vi "NernstIV.vi"() -> ()   [LabVIEW 2020]
uses:
  <userlib>/LevyLab/LV-Data/LV-Data/Typedefs/Dictionary--cluster.ctl
  <userlib>/LevyLab/LV-Data/LV-Data/Typedefs/File Type--enum.ctl
  <userlib>/LevyLab/XY Utilities/subVIs/Subtract XY (single).vi
  <userlib>/LevyLab/XY Utilities/subVIs/Moving Average (single).vi
  <userlib>/LevyLab/XY Utilities/subVIs/Get X and Y (single).vi
  <userlib>/LevyLab/XY Utilities/Private/X Units.vi
  <userlib>/LevyLab/XY Utilities/Private/X Array Range to Index.vi
  <userlib>/_OpenG.lib/array/array.llb/Sort Array__ogtk.vi
  <userlib>/_OpenG.lib/array/array.llb/Sort 1D Array (DBL)__ogtk.vi
  <userlib>/_OpenG.lib/array/array.llb/Reorder Array2__ogtk.vi
  <userlib>/_OpenG.lib/array/array.llb/Reorder 1D Array2 (DBL)__ogtk.vi
  <vilib>/ptbypt/Probability & Statistics.llb/Mean PtByPt.vi
  <vilib>/Utility/error.llb/Error Cluster From Error Code.vi
  <userlib>/LevyLab/LV-Data/LV-Data/LV-Data.lvclass
  <userlib>/LevyLab/XY Utilities/xy_utilities.lvlib
panel:
  in  "Avg Window":dbl
  out "Error vs Temp 2T":cluster{dbl[], dbl[]}[](graph)=[{[0.099648], [2.4953013324737623e-06]}]
  in  "Antisym?":bool
  in  "length per file":i32=196
  in  "index":i32=99
  out "Error vs Temp":cluster{dbl[], dbl[]}[](graph)=[{[0.099648], [0.0]}]
  in  "File Type":T1=enum."TDMS"
  out "counter":i32
  out "Path":path=path "G:/.shortcut-targets-by-id/0B8-gGFa6hkR4XzJJMDlqZXVKRk0/ansom/Data/PPMS 3/SA40511C.20250205/08-IVWire1nd2_heating/SA40511C.20250205.000008.tdms"
  out "Comments":string="Device: \r  Device Name: SA40511C.20250205\r  Computer: PPMS3DAQ\r  User: Ranjani\r  Instrument: PPMS 3\r  Description: |\r    LAO/KTO 3wire Nernst\r\rExperiment: \r  Time: 2025-02-08T20:02:05\r  Description: |\r    T =100mK\r    B= 1T\r    \r    I1 and 2+= 0 to -50m to 50m to 0V, 30s\r    wait, 2s\r    I+/- = 2/5\r    V+/- = 1/26\r    I2+/- = 3/4\r    Wire 3\r    I3+/- =100 mV @13Hz (346nA)\r\rSweep: \r- Loop1: [OFF, 0.000000]\r- Loop2: [OFF, 0.000000]\r- Loop3: [OFF, 0.000000]\r- Loop4: [OFF, 0.000000]\r\rWiring: \r- Electrode 1: Lockin 1, V1+\r- Electrode 2: Lockin 2, I+\r- Electrode 3: Lockin 3, I2+\r- Electrode 4: Lockin 4, I2-\r- Electrode 5: Lockin 5, I-\r- Electrode 26: Lockin 6, V1-\r- Electrode 27: Lockin 7, I3+\r- Electrode 28: Lockin 8, I3+\r\rLockin: \r  AO: \r  - AO 1: amp = 0.000 mV, DC = 0.000 mV, f = 13.00 Hz, phi = 0.00°, Sine\r  - AO 2: amp = 0.000 mV, DC = 0.001 mV, f = 13.00 Hz, phi = 0.00°, Sine\r  - AO 3: amp = 0.000 mV, DC = 0.001 mV, f = 13.00 Hz, phi = 0.00°, Sine\r  - AO 4: amp = 0.000 mV, DC = 0.000 mV, f = 13.00 Hz, phi = 0.00°, Sine\r  - AO 5: amp = 0.000 mV, DC = 0.000 mV, f = 13.00 Hz, phi = 0.00°, Sine\r  - AO 6: amp = 0.000 mV, DC = 0.000 mV, f = 13.00 Hz, phi = 0.00°, Sine\r  - AO 7: amp = 0.000 mV, DC = 0.000 mV, f = 13.00 Hz, phi = 0.00°, Sine\r  - AO 8: amp = 100.000 mV, DC = 0.000 mV, f = 13.00 Hz, phi = 0.00°, Sine\r  REF: \r  - Lockin 1: f = 13.00 Hz, phi = 0.00°, TC = 0.10 s, order = 2 \r  - Lockin 2: f = 26.00 Hz, phi = 0.00°, TC = 0.10 s, order = 2 \r  Sampling: \r  - Fs: 13000.000000\r  - N: 1000\r"
  in  "index":T2={"I+(A)"="AO2", "I-(A)"="AI5", "V4T+"="AI1", "V4T-"="AI6", "UG"="AO3", "DG"="AO4", "LG"="AO8", "B"="Magnet", "Temperature"="Temperature", "Vfast"="Temperature", "Vslow"="Magnet"}
  in  "SE?":bool=TRUE
  out "Data (Dictionary)":T3[](array[typedef])=[{"key"="Time", "value"=variant(dbl[] [3821910664.275333])}, {"key"="Temperature", "value"=variant(dbl[] [0.099648])}, {"key"="Magnet", "value"=variant(dbl[] [0.99993349609375])}, {"key"="AO1", "value"=variant(dbl[] [0.0, 0.0, 0.0, 0.0, 0.0, 0.0, 0.0, 0.0, 0.0, 0.0, 0.0, 0.0, 0.0, 0.0, 0.0, 0.0, 0.0, 0.0, 0.0, 0.0, 0.0, 0.0, 0.0, 0.0, 0.0, 0.0, 0.0, 0.0, 0.0, 0.0, 0.0, 0.0, 0.0, 0.0, 0.0, 0.0, 0.0, 0.0, 0.0, 0.0, 0.0, 0.0, 0.0, 0.0, 0.0, 0.0, 0.0, 0.0, 0.0, 0.0, 0.0, 0.0, 0.0, 0.0, 0.0, 0.0, 0.0, 0.0, 0.0, 0.0, 0.0, 0.0, 0.0, 0.0, 0.0, 0.0, 0.0, 0.0, 0.0, 0.0, 0.0, 0.0, 0.0, 0.0, 0.0, 0.0, 0.0, 0.0, 0.0, 0.0, 0.0, 0.0, 0.0, 0.0, 0.0, 0.0, 0.0, 0.0, 0.0, 0.0, 0.0, 0.0, 0.0, 0.0, 0.0, 0.0, 0.0, 0.0, 0.0, 0.0, 0.0, 0.0, 0.0, 0.0, 0.0, 0.0, 0.0, 0.0, 0.0, 0.0, 0.0, 0.0, 0.0, 0.0, 0.0, 0.0, 0.0, 0.0, 0.0, 0.0, 0.0, 0.0, 0.0, 0.0, 0.0, 0.0, 0.0, 0.0, 0.0, 0.0, 0.0, 0.0, 0.0, 0.0, 0.0, 0.0, 0.0, 0.0, 0.0, 0.0, 0.0, 0.0, 0.0, 0.0, 0.0, 0.0, 0.0, 0.0, 0.0, 0.0, 0.0, 0.0, 0.0, 0.0, 0.0, 0.0, 0.0, 0.0, 0.0, 0.0, 0.0, 0.0, 0.0, 0.0, 0.0, 0.0, 0.0, 0.0, 0.0, 0.0, 0.0, 0.0, 0.0, 0.0, 0.0, 0.0, 0.0, 0.0, 0.0, 0.0, 0.0, 0.0, 0.0, 0.0, 0.0, 0.0, 0.0, 0.0, 0.0, 0.0, 0.0, 0.0, 0.0, 0.0, 0.0, 0.0, 0.0, 0.0, 0.0, 0.0, 0.0, 0.0, 0.0, 0.0, 0.0, 0.0, 0.0, 0.0, 0.0, 0.0, 0.0, 0.0, 0.0, 0.0, 0.0, 0.0, 0.0, 0.0, 0.0, 0.0, 0.0, 0.0, 0.0, 0.0, 0.0, 0.0, 0.0, 0.0, 0.0, 0.0, 0.0, 0.0, 0.0, 0.0, 0.0, 0.0, 0.0, 0.0, 0.0, 0.0, 0.0, 0.0, 0.0, 0.0, 0.0, 0.0, 0.0, 0.0, 0.0, 0.0, 0.0, 0.0, 0.0, 0.0, 0.0, 0.0, 0.0, 0.0, 0.0, 0.0, 0.0, 0.0, 0.0, 0.0, 0.0, 0.0, 0.0, 0.0, 0.0, 0.0, 0.0, 0.0, 0.0, 0.0, 0.0, 0.0, 0.0, 0.0, 0.0, 0.0, 0.0, 0.0, 0.0, 0.0, 0.0, 0.0, 0.0, 0.0, 0.0, 0.0, 0.0, 0.0, 0.0, 0.0, 0.0, 0.0, 0.0, 0.0, 0.0, 0.0, 0.0, 0.0, 0.0, 0.0, 0.0, 0.0, 0.0, 0.0, 0.0, 0.0, 0.0, 0.0, 0.0, 0.0, 0.0, 0.0, 0.0, 0.0, 0.0, 0.0, 0.0, 0.0, 0.0, 0.0, 0.0, 0.0, 0.0, 0.0, 0.0, 0.0, 0.0, 0.0, 0.0, 0.0, 0.0, 0.0, 0.0, 0.0, 0.0, 0.0, 0.0, 0.0, 0.0, 0.0, 0.0, 0.0, 0.0, 0.0, 0.0, 0.0, 0.0, 0.0, 0.0, 0.0, 0.0, 0.0, 0.0, 0.0, 0.0, 0.0, 0.0, 0.0, 0.0, 0.0, 0.0, 0.0, 0.0, 0.0, 0.0, 0.0, 0.0, 0.0, 0.0, 0.0, 0.0, 0.0, 0.0, 0.0, 0.0, 0.0, 0.0, 0.0, 0.0, 0.0, 0.0, 0.0, 0.0, 0.0, 0.0, 0.0])}, {"key"="AO2", "value"=variant(dbl[] array[390 elements])}, {"key"="AO3", "value"=variant(dbl[] array[390 elements])}, {"key"="AO4", "value"=variant(dbl[] [0.0, 0.0, 0.0, 0.0, 0.0, 0.0, 0.0, 0.0, 0.0, 0.0, 0.0, 0.0, 0.0, 0.0, 0.0, 0.0, 0.0, 0.0, 0.0, 0.0, 0.0, 0.0, 0.0, 0.0, 0.0, 0.0, 0.0, 0.0, 0.0, 0.0, 0.0, 0.0, 0.0, 0.0, 0.0, 0.0, 0.0, 0.0, 0.0, 0.0, 0.0, 0.0, 0.0, 0.0, 0.0, 0.0, 0.0, 0.0, 0.0, 0.0, 0.0, 0.0, 0.0, 0.0, 0.0, 0.0, 0.0, 0.0, 0.0, 0.0, 0.0, 0.0, 0.0, 0.0, 0.0, 0.0, 0.0, 0.0, 0.0, 0.0, 0.0, 0.0, 0.0, 0.0, 0.0, 0.0, 0.0, 0.0, 0.0, 0.0, 0.0, 0.0, 0.0, 0.0, 0.0, 0.0, 0.0, 0.0, 0.0, 0.0, 0.0, 0.0, 0.0, 0.0, 0.0, 0.0, 0.0, 0.0, 0.0, 0.0, 0.0, 0.0, 0.0, 0.0, 0.0, 0.0, 0.0, 0.0, 0.0, 0.0, 0.0, 0.0, 0.0, 0.0, 0.0, 0.0, 0.0, 0.0, 0.0, 0.0, 0.0, 0.0, 0.0, 0.0, 0.0, 0.0, 0.0, 0.0, 0.0, 0.0, 0.0, 0.0, 0.0, 0.0, 0.0, 0.0, 0.0, 0.0, 0.0, 0.0, 0.0, 0.0, 0.0, 0.0, 0.0, 0.0, 0.0, 0.0, 0.0, 0.0, 0.0, 0.0, 0.0, 0.0, 0.0, 0.0, 0.0, 0.0, 0.0, 0.0, 0.0, 0.0, 0.0, 0.0, 0.0, 0.0, 0.0, 0.0, 0.0, 0.0, 0.0, 0.0, 0.0, 0.0, 0.0, 0.0, 0.0, 0.0, 0.0, 0.0, 0.0, 0.0, 0.0, 0.0, 0.0, 0.0, 0.0, 0.0, 0.0, 0.0, 0.0, 0.0, 0.0, 0.0, 0.0, 0.0, 0.0, 0.0, 0.0, 0.0, 0.0, 0.0, 0.0, 0.0, 0.0, 0.0, 0.0, 0.0, 0.0, 0.0, 0.0, 0.0, 0.0, 0.0, 0.0, 0.0, 0.0, 0.0, 0.0, 0.0, 0.0, 0.0, 0.0, 0.0, 0.0, 0.0, 0.0, 0.0, 0.0, 0.0, 0.0, 0.0, 0.0, 0.0, 0.0, 0.0, 0.0, 0.0, 0.0, 0.0, 0.0, 0.0, 0.0, 0.0, 0.0, 0.0, 0.0, 0.0, 0.0, 0.0, 0.0, 0.0, 0.0, 0.0, 0.0, 0.0, 0.0, 0.0, 0.0, 0.0, 0.0, 0.0, 0.0, 0.0, 0.0, 0.0, 0.0, 0.0, 0.0, 0.0, 0.0, 0.0, 0.0, 0.0, 0.0, 0.0, 0.0, 0.0, 0.0, 0.0, 0.0, 0.0, 0.0, 0.0, 0.0, 0.0, 0.0, 0.0, 0.0, 0.0, 0.0, 0.0, 0.0, 0.0, 0.0, 0.0, 0.0, 0.0, 0.0, 0.0, 0.0, 0.0, 0.0, 0.0, 0.0, 0.0, 0.0, 0.0, 0.0, 0.0, 0.0, 0.0, 0.0, 0.0, 0.0, 0.0, 0.0, 0.0, 0.0, 0.0, 0.0, 0.0, 0.0, 0.0, 0.0, 0.0, 0.0, 0.0, 0.0, 0.0, 0.0, 0.0, 0.0, 0.0, 0.0, 0.0, 0.0, 0.0, 0.0, 0.0, 0.0, 0.0, 0.0, 0.0, 0.0, 0.0, 0.0, 0.0, 0.0, 0.0, 0.0, 0.0, 0.0, 0.0, 0.0, 0.0, 0.0, 0.0, 0.0, 0.0, 0.0, 0.0, 0.0, 0.0, 0.0, 0.0, 0.0, 0.0, 0.0, 0.0, 0.0, 0.0, 0.0, 0.0, 0.0, 0.0, 0.0, 0.0, 0.0, 0.0, 0.0, 0.0, 0.0, 0.0, 0.0, 0.0, 0.0, 0.0, 0.0, 0.0])}, {"key"="AO5", "value"=variant(dbl[] [0.0, 0.0, 0.0, 0.0, 0.0, 0.0, 0.0, 0.0, 0.0, 0.0, 0.0, 0.0, 0.0, 0.0, 0.0, 0.0, 0.0, 0.0, 0.0, 0.0, 0.0, 0.0, 0.0, 0.0, 0.0, 0.0, 0.0, 0.0, 0.0, 0.0, 0.0, 0.0, 0.0, 0.0, 0.0, 0.0, 0.0, 0.0, 0.0, 0.0, 0.0, 0.0, 0.0, 0.0, 0.0, 0.0, 0.0, 0.0, 0.0, 0.0, 0.0, 0.0, 0.0, 0.0, 0.0, 0.0, 0.0, 0.0, 0.0, 0.0, 0.0, 0.0, 0.0, 0.0, 0.0, 0.0, 0.0, 0.0, 0.0, 0.0, 0.0, 0.0, 0.0, 0.0, 0.0, 0.0, 0.0, 0.0, 0.0, 0.0, 0.0, 0.0, 0.0, 0.0, 0.0, 0.0, 0.0, 0.0, 0.0, 0.0, 0.0, 0.0, 0.0, 0.0, 0.0, 0.0, 0.0, 0.0, 0.0, 0.0, 0.0, 0.0, 0.0, 0.0, 0.0, 0.0, 0.0, 0.0, 0.0, 0.0, 0.0, 0.0, 0.0, 0.0, 0.0, 0.0, 0.0, 0.0, 0.0, 0.0, 0.0, 0.0, 0.0, 0.0, 0.0, 0.0, 0.0, 0.0, 0.0, 0.0, 0.0, 0.0, 0.0, 0.0, 0.0, 0.0, 0.0, 0.0, 0.0, 0.0, 0.0, 0.0, 0.0, 0.0, 0.0, 0.0, 0.0, 0.0, 0.0, 0.0, 0.0, 0.0, 0.0, 0.0, 0.0, 0.0, 0.0, 0.0, 0.0, 0.0, 0.0, 0.0, 0.0, 0.0, 0.0, 0.0, 0.0, 0.0, 0.0, 0.0, 0.0, 0.0, 0.0, 0.0, 0.0, 0.0, 0.0, 0.0, 0.0, 0.0, 0.0, 0.0, 0.0, 0.0, 0.0, 0.0, 0.0, 0.0, 0.0, 0.0, 0.0, 0.0, 0.0, 0.0, 0.0, 0.0, 0.0, 0.0, 0.0, 0.0, 0.0, 0.0, 0.0, 0.0, 0.0, 0.0, 0.0, 0.0, 0.0, 0.0, 0.0, 0.0, 0.0, 0.0, 0.0, 0.0, 0.0, 0.0, 0.0, 0.0, 0.0, 0.0, 0.0, 0.0, 0.0, 0.0, 0.0, 0.0, 0.0, 0.0, 0.0, 0.0, 0.0, 0.0, 0.0, 0.0, 0.0, 0.0, 0.0, 0.0, 0.0, 0.0, 0.0, 0.0, 0.0, 0.0, 0.0, 0.0, 0.0, 0.0, 0.0, 0.0, 0.0, 0.0, 0.0, 0.0, 0.0, 0.0, 0.0, 0.0, 0.0, 0.0, 0.0, 0.0, 0.0, 0.0, 0.0, 0.0, 0.0, 0.0, 0.0, 0.0, 0.0, 0.0, 0.0, 0.0, 0.0, 0.0, 0.0, 0.0, 0.0, 0.0, 0.0, 0.0, 0.0, 0.0, 0.0, 0.0, 0.0, 0.0, 0.0, 0.0, 0.0, 0.0, 0.0, 0.0, 0.0, 0.0, 0.0, 0.0, 0.0, 0.0, 0.0, 0.0, 0.0, 0.0, 0.0, 0.0, 0.0, 0.0, 0.0, 0.0, 0.0, 0.0, 0.0, 0.0, 0.0, 0.0, 0.0, 0.0, 0.0, 0.0, 0.0, 0.0, 0.0, 0.0, 0.0, 0.0, 0.0, 0.0, 0.0, 0.0, 0.0, 0.0, 0.0, 0.0, 0.0, 0.0, 0.0, 0.0, 0.0, 0.0, 0.0, 0.0, 0.0, 0.0, 0.0, 0.0, 0.0, 0.0, 0.0, 0.0, 0.0, 0.0, 0.0, 0.0, 0.0, 0.0, 0.0, 0.0, 0.0, 0.0, 0.0, 0.0, 0.0, 0.0, 0.0, 0.0, 0.0, 0.0, 0.0, 0.0, 0.0, 0.0, 0.0, 0.0, 0.0, 0.0, 0.0, 0.0, 0.0, 0.0, 0.0, 0.0, 0.0, 0.0, 0.0, 0.0, 0.0, 0.0])}, {"key"="AO6", "value"=variant(dbl[] [0.0, 0.0, 0.0, 0.0, 0.0, 0.0, 0.0, 0.0, 0.0, 0.0, 0.0, 0.0, 0.0, 0.0, 0.0, 0.0, 0.0, 0.0, 0.0, 0.0, 0.0, 0.0, 0.0, 0.0, 0.0, 0.0, 0.0, 0.0, 0.0, 0.0, 0.0, 0.0, 0.0, 0.0, 0.0, 0.0, 0.0, 0.0, 0.0, 0.0, 0.0, 0.0, 0.0, 0.0, 0.0, 0.0, 0.0, 0.0, 0.0, 0.0, 0.0, 0.0, 0.0, 0.0, 0.0, 0.0, 0.0, 0.0, 0.0, 0.0, 0.0, 0.0, 0.0, 0.0, 0.0, 0.0, 0.0, 0.0, 0.0, 0.0, 0.0, 0.0, 0.0, 0.0, 0.0, 0.0, 0.0, 0.0, 0.0, 0.0, 0.0, 0.0, 0.0, 0.0, 0.0, 0.0, 0.0, 0.0, 0.0, 0.0, 0.0, 0.0, 0.0, 0.0, 0.0, 0.0, 0.0, 0.0, 0.0, 0.0, 0.0, 0.0, 0.0, 0.0, 0.0, 0.0, 0.0, 0.0, 0.0, 0.0, 0.0, 0.0, 0.0, 0.0, 0.0, 0.0, 0.0, 0.0, 0.0, 0.0, 0.0, 0.0, 0.0, 0.0, 0.0, 0.0, 0.0, 0.0, 0.0, 0.0, 0.0, 0.0, 0.0, 0.0, 0.0, 0.0, 0.0, 0.0, 0.0, 0.0, 0.0, 0.0, 0.0, 0.0, 0.0, 0.0, 0.0, 0.0, 0.0, 0.0, 0.0, 0.0, 0.0, 0.0, 0.0, 0.0, 0.0, 0.0, 0.0, 0.0, 0.0, 0.0, 0.0, 0.0, 0.0, 0.0, 0.0, 0.0, 0.0, 0.0, 0.0, 0.0, 0.0, 0.0, 0.0, 0.0, 0.0, 0.0, 0.0, 0.0, 0.0, 0.0, 0.0, 0.0, 0.0, 0.0, 0.0, 0.0, 0.0, 0.0, 0.0, 0.0, 0.0, 0.0, 0.0, 0.0, 0.0, 0.0, 0.0, 0.0, 0.0, 0.0, 0.0, 0.0, 0.0, 0.0, 0.0, 0.0, 0.0, 0.0, 0.0, 0.0, 0.0, 0.0, 0.0, 0.0, 0.0, 0.0, 0.0, 0.0, 0.0, 0.0, 0.0, 0.0, 0.0, 0.0, 0.0, 0.0, 0.0, 0.0, 0.0, 0.0, 0.0, 0.0, 0.0, 0.0, 0.0, 0.0, 0.0, 0.0, 0.0, 0.0, 0.0, 0.0, 0.0, 0.0, 0.0, 0.0, 0.0, 0.0, 0.0, 0.0, 0.0, 0.0, 0.0, 0.0, 0.0, 0.0, 0.0, 0.0, 0.0, 0.0, 0.0, 0.0, 0.0, 0.0, 0.0, 0.0, 0.0, 0.0, 0.0, 0.0, 0.0, 0.0, 0.0, 0.0, 0.0, 0.0, 0.0, 0.0, 0.0, 0.0, 0.0, 0.0, 0.0, 0.0, 0.0, 0.0, 0.0, 0.0, 0.0, 0.0, 0.0, 0.0, 0.0, 0.0, 0.0, 0.0, 0.0, 0.0, 0.0, 0.0, 0.0, 0.0, 0.0, 0.0, 0.0, 0.0, 0.0, 0.0, 0.0, 0.0, 0.0, 0.0, 0.0, 0.0, 0.0, 0.0, 0.0, 0.0, 0.0, 0.0, 0.0, 0.0, 0.0, 0.0, 0.0, 0.0, 0.0, 0.0, 0.0, 0.0, 0.0, 0.0, 0.0, 0.0, 0.0, 0.0, 0.0, 0.0, 0.0, 0.0, 0.0, 0.0, 0.0, 0.0, 0.0, 0.0, 0.0, 0.0, 0.0, 0.0, 0.0, 0.0, 0.0, 0.0, 0.0, 0.0, 0.0, 0.0, 0.0, 0.0, 0.0, 0.0, 0.0, 0.0, 0.0, 0.0, 0.0, 0.0, 0.0, 0.0, 0.0, 0.0, 0.0, 0.0, 0.0, 0.0, 0.0, 0.0, 0.0, 0.0, 0.0, 0.0, 0.0, 0.0, 0.0, 0.0, 0.0, 0.0])}, {"key"="AO7", "value"=variant(dbl[] [0.0, 0.0, 0.0, 0.0, 0.0, 0.0, 0.0, 0.0, 0.0, 0.0, 0.0, 0.0, 0.0, 0.0, 0.0, 0.0, 0.0, 0.0, 0.0, 0.0, 0.0, 0.0, 0.0, 0.0, 0.0, 0.0, 0.0, 0.0, 0.0, 0.0, 0.0, 0.0, 0.0, 0.0, 0.0, 0.0, 0.0, 0.0, 0.0, 0.0, 0.0, 0.0, 0.0, 0.0, 0.0, 0.0, 0.0, 0.0, 0.0, 0.0, 0.0, 0.0, 0.0, 0.0, 0.0, 0.0, 0.0, 0.0, 0.0, 0.0, 0.0, 0.0, 0.0, 0.0, 0.0, 0.0, 0.0, 0.0, 0.0, 0.0, 0.0, 0.0, 0.0, 0.0, 0.0, 0.0, 0.0, 0.0, 0.0, 0.0, 0.0, 0.0, 0.0, 0.0, 0.0, 0.0, 0.0, 0.0, 0.0, 0.0, 0.0, 0.0, 0.0, 0.0, 0.0, 0.0, 0.0, 0.0, 0.0, 0.0, 0.0, 0.0, 0.0, 0.0, 0.0, 0.0, 0.0, 0.0, 0.0, 0.0, 0.0, 0.0, 0.0, 0.0, 0.0, 0.0, 0.0, 0.0, 0.0, 0.0, 0.0, 0.0, 0.0, 0.0, 0.0, 0.0, 0.0, 0.0, 0.0, 0.0, 0.0, 0.0, 0.0, 0.0, 0.0, 0.0, 0.0, 0.0, 0.0, 0.0, 0.0, 0.0, 0.0, 0.0, 0.0, 0.0, 0.0, 0.0, 0.0, 0.0, 0.0, 0.0, 0.0, 0.0, 0.0, 0.0, 0.0, 0.0, 0.0, 0.0, 0.0, 0.0, 0.0, 0.0, 0.0, 0.0, 0.0, 0.0, 0.0, 0.0, 0.0, 0.0, 0.0, 0.0, 0.0, 0.0, 0.0, 0.0, 0.0, 0.0, 0.0, 0.0, 0.0, 0.0, 0.0, 0.0, 0.0, 0.0, 0.0, 0.0, 0.0, 0.0, 0.0, 0.0, 0.0, 0.0, 0.0, 0.0, 0.0, 0.0, 0.0, 0.0, 0.0, 0.0, 0.0, 0.0, 0.0, 0.0, 0.0, 0.0, 0.0, 0.0, 0.0, 0.0, 0.0, 0.0, 0.0, 0.0, 0.0, 0.0, 0.0, 0.0, 0.0, 0.0, 0.0, 0.0, 0.0, 0.0, 0.0, 0.0, 0.0, 0.0, 0.0, 0.0, 0.0, 0.0, 0.0, 0.0, 0.0, 0.0, 0.0, 0.0, 0.0, 0.0, 0.0, 0.0, 0.0, 0.0, 0.0, 0.0, 0.0, 0.0, 0.0, 0.0, 0.0, 0.0, 0.0, 0.0, 0.0, 0.0, 0.0, 0.0, 0.0, 0.0, 0.0, 0.0, 0.0, 0.0, 0.0, 0.0, 0.0, 0.0, 0.0, 0.0, 0.0, 0.0, 0.0, 0.0, 0.0, 0.0, 0.0, 0.0, 0.0, 0.0, 0.0, 0.0, 0.0, 0.0, 0.0, 0.0, 0.0, 0.0, 0.0, 0.0, 0.0, 0.0, 0.0, 0.0, 0.0, 0.0, 0.0, 0.0, 0.0, 0.0, 0.0, 0.0, 0.0, 0.0, 0.0, 0.0, 0.0, 0.0, 0.0, 0.0, 0.0, 0.0, 0.0, 0.0, 0.0, 0.0, 0.0, 0.0, 0.0, 0.0, 0.0, 0.0, 0.0, 0.0, 0.0, 0.0, 0.0, 0.0, 0.0, 0.0, 0.0, 0.0, 0.0, 0.0, 0.0, 0.0, 0.0, 0.0, 0.0, 0.0, 0.0, 0.0, 0.0, 0.0, 0.0, 0.0, 0.0, 0.0, 0.0, 0.0, 0.0, 0.0, 0.0, 0.0, 0.0, 0.0, 0.0, 0.0, 0.0, 0.0, 0.0, 0.0, 0.0, 0.0, 0.0, 0.0, 0.0, 0.0, 0.0, 0.0, 0.0, 0.0, 0.0, 0.0, 0.0, 0.0, 0.0, 0.0, 0.0, 0.0, 0.0, 0.0, 0.0, 0.0, 0.0, 0.0])}, {"key"="AO8", "value"=variant(dbl[] array[390 elements])}, {"key"="AI1", "value"=variant(dbl[] array[390 elements])}, {"key"="AI2", "value"=variant(dbl[] array[390 elements])}, {"key"="AI3", "value"=variant(dbl[] array[390 elements])}, {"key"="AI4", "value"=variant(dbl[] array[390 elements])}, {"key"="AI5", "value"=variant(dbl[] array[390 elements])}, {"key"="AI6", "value"=variant(dbl[] array[390 elements])}, {"key"="AI7", "value"=variant(dbl[] array[390 elements])}, {"key"="AI8", "value"=variant(dbl[] array[390 elements])}, {"key"="X1", "value"=variant(dbl[] array[390 elements])}, {"key"="X2", "value"=variant(dbl[] array[390 elements])}, {"key"="X3", "value"=variant(dbl[] array[390 elements])}, {"key"="X4", "value"=variant(dbl[] array[390 elements])}, {"key"="X5", "value"=variant(dbl[] array[390 elements])}, {"key"="X6", "value"=variant(dbl[] array[390 elements])}, {"key"="X7", "value"=variant(dbl[] array[390 elements])}, {"key"="X8", "value"=variant(dbl[] array[390 elements])}, {"key"="Y1", "value"=variant(dbl[] array[390 elements])}, {"key"="Y2", "value"=variant(dbl[] array[390 elements])}, {"key"="Y3", "value"=variant(dbl[] array[390 elements])}, {"key"="Y4", "value"=variant(dbl[] array[390 elements])}, {"key"="Y5", "value"=variant(dbl[] array[390 elements])}, {"key"="Y6", "value"=variant(dbl[] array[390 elements])}, {"key"="Y7", "value"=variant(dbl[] array[390 elements])}, {"key"="Y8", "value"=variant(dbl[] array[390 elements])}]
  out "Gates, B and T":T4={"UG"=-0.000255897435897436, "DG"=0.0, "LG"=7.77808822991638e-13, "B"=0.99993349609375, "Temperature"=0.099648}
  in  "Subtract from 4T":cluster{dbl[], dbl[]}[](graph)=[{[-0.020298805594444295, -0.020143332123756498, -0.019935172677040203, -0.019711892008781505, -0.019499069094658004, -0.019296326518058897, -0.0190861269235612, -0.018870721936226, -0.0186526147127153, -0.0184441012144091, -0.018240182995796404, -0.018026167988777403, -0.017805154204368796, -0.0175968400239946, -0.017388032078743197, -0.017181379437446798, -0.016960291981697302, -0.016742527604103302, -0.0165384343862536, -0.0163279012441638, -0.0161165035963061, -0.0158924008607867, -0.0156821869611742, -0.015477146983146901, -0.015263935208320902, -0.0150432082414629, -0.014828914046287701, -0.0146212004423143, -0.0144141832590105, -0.0141964107751848, -0.0139734686613085, -0.013768090128898802, -0.0135563558340074, -0.013346166729927202, -0.013120899081230299, -0.0129057987928392, -0.012701104283332999, -0.012487238287925912, -0.01226870453357717, -0.01204702484607715, -0.01183656013011947, -0.01162859666347524, -0.01141238462924974, -0.01118832433223746, -0.010975580811500699, -0.01076415216922773, -0.010553850293159662, -0.010330365061760138, -0.010109158396721092, -0.009902112841606301, -0.00968768084049235, -0.00947194325923932, -0.009244939923286621, -0.009032684683799868, -0.00882454001903547, -0.00860845100879677, -0.00838605582714088, -0.008168872952461409, -0.00795692384243022, -0.007747506260871981, -0.007525480151176509, -0.007301862120628491, -0.007093491911888181, -0.0068792678117752595, -0.0066681920289994095, -0.00644138252735143, -0.0062280436754227, -0.00602158486843118, -0.005808955550193789, -0.00559199845790865, -0.00537080562114718, -0.005163264632225051, -0.0049578579664230306, -0.00474451506137847, -0.004523096442222571, -0.004317351222038229, -0.0041118384599685195, -0.0039091233015059994, -0.00369388210773464, -0.0034842001199722, -0.0032883435487746897, -0.0030877457857131797, -0.0028865646123886, -0.0026763523817062403, -0.00248287928104402, -0.0022957037687301902, -0.0021012431383133304, -0.0018998574018478898, -0.00170761549472813, -0.0015246480703354297, -0.0013457845449447899, -0.0011569598913192998, -0.0009671784639358609, -0.000797939419746412, -0.0006248732805252139, -0.00045578753948211396, -0.00027331769466399497, -0.00010534942150116299, 4.9853920936584e-05, 0.00021248924732208502, 0.00038257944583893004, 0.000559727311134333, 0.000726794123649592, 0.000892312169075, 0.00107245266437529, 0.0012648783922195202, 0.00144211494922634, 0.00162198793888088, 0.0018035722970962, 0.00200244796276088, 0.0021988219022750504, 0.0023840004205703496, 0.00257733285427093, 0.0027730993032455404, 0.00298340857028962, 0.00318200647830965, 0.0033764384984970304, 0.00358172023296359, 0.0037975507974625003, 0.00400608170032506, 0.004211035609245349, 0.00441424405574801, 0.00463290369510651, 0.004853630900382989, 0.00505880463123321, 0.00527102982997892, 0.00548183524608609, 0.00570913612842555, 0.0059262028932570805, 0.0061337746381759, 0.006350606799125561, 0.00657308328151695, 0.006797502160072209, 0.00701170980930318, 0.007223751902580171, 0.007445839762687629, 0.0076745249032973495, 0.00788892495632163, 0.008105991482734609, 0.00832066643238058, 0.00854929745197286, 0.008773327469825608, 0.008985962748527383, 0.009204881548881421, 0.00942662870883931, 0.009656422495841838, 0.009873687624931172, 0.01008750140666952, 0.010308032870292512, 0.010535851359367219, 0.010755051493644521, 0.01097254836559275, 0.011186535954475272, 0.01141592419147475, 0.01164573872089373, 0.01185890591144548, 0.01207890450954417, 0.01229698598384842, 0.0125287271738051, 0.012748497128486448, 0.012961129307746701, 0.0131815141439436, 0.0134082280397413, 0.013634177565574501, 0.0138529192209242, 0.014067153573036, 0.014290386795997399, 0.0145212532281873, 0.0147375079393385, 0.014956275105476199, 0.015173210740089201, 0.0154038113355635, 0.0156266974210737, 0.0158396693468092, 0.016059869408607298, 0.0162831009626387, 0.0165129681825636, 0.0167303055524824, 0.016944220423698197, 0.0171680797338483, 0.0173991161584852, 0.017618041872978, 0.017834319472312697, 0.018048580527305402, 0.0182773231267927, 0.018506924033164802, 0.0187209612131117, 0.018940549969673003, 0.0191605340242385, 0.019393757939338598, 0.019613784909248304, 0.0198268069028853, 0.0200480521917343, 0.020275678992271395, 0.0205016232728957, 0.0206638196706772], [-1.88530516624451e-07, -1.87133288383484e-07, -1.85253167152405e-07, -1.83320441246033e-07, -1.81518726348877e-07, -1.79542255401611e-07, -1.77687950134277e-07, -1.75797801017761e-07, -1.73898572921753e-07, -1.71995229721069e-07, -1.70092630386353e-07, -1.68203616142273e-07, -1.6635901927948e-07, -1.64455137252808e-07, -1.62550988197327e-07, -1.60638189315796e-07, -1.58735628128052e-07, -1.56911063194275e-07, -1.54978852272034e-07, -1.53096804618836e-07, -1.51216950416565e-07, -1.49291834831238e-07, -1.47456007003784e-07, -1.45557689666748e-07, -1.4364326953888e-07, -1.41811571121216e-07, -1.3987343788147e-07, -1.38007555007935e-07, -1.36112055778503e-07, -1.34210629463196e-07, -1.3238597869873e-07, -1.30467686653137e-07, -1.28578906059265e-07, -1.26701898574829e-07, -1.24821209907532e-07, -1.22998299598694e-07, -1.21071562767029e-07, -1.19200682640076e-07, -1.17325396537781e-07, -1.15441784858704e-07, -1.1358193397522e-07, -1.11678218841553e-07, -1.09816336631775e-07, -1.0796443939209e-07, -1.06044731140137e-07, -1.04197044372559e-07, -1.02285056114197e-07, -1.00400342941284e-07, -9.85824632644653e-08, -9.66873502731323e-08, -9.47991418838502e-08, -9.29165840148925e-08, -9.10269689559937e-08, -8.91835737228393e-08, -8.72648000717163e-08, -8.53948640823364e-08, -8.35837936401368e-08, -8.16421175003052e-08, -7.9793062210083e-08, -7.79200601577759e-08, -7.59902238845825e-08, -7.42254400253296e-08, -7.22940492630005e-08, -7.04062414169312e-08, -6.84745645523071e-08, -6.65928602218628e-08, -6.47673559188843e-08, -6.28309917449951e-08, -6.0914454460144e-08, -5.90352773666382e-08, -5.7114372253418e-08, -5.52046394348144e-08, -5.32772445678711e-08, -5.13371229171753e-08, -4.94526720046997e-08, -4.74649143218994e-08, -4.55275678634644e-08, -4.35710477828979e-08, -4.159517288208e-08, -3.96825170516968e-08, -3.76472520828247e-08, -3.56490802764893e-08, -3.36032581329346e-08, -3.15900993347168e-08, -2.95552396774292e-08, -2.74624919891357e-08, -2.53818082809448e-08, -2.33121252059936e-08, -2.11334800720215e-08, -1.90311288833618e-08, -1.68199777603149e-08, -1.46402263641357e-08, -1.24739789962768e-08, -1.02206993103027e-08, -7.93179988861084e-09, -5.64008235931397e-09, -3.30891609191894e-09, -1.04283332824707e-09, 1.40513420104981e-09, 3.84415149688721e-09, 6.134033203125e-09, 8.53836059570313e-09, 1.08101654052734e-08, 1.31109428405762e-08, 1.53783369064331e-08, 1.75216150283813e-08, 1.97556734085083e-08, 2.19318246841431e-08, 2.40856266021728e-08, 2.62651681900024e-08, 2.82614612579346e-08, 3.04032325744629e-08, 3.24541425704956e-08, 3.45364236831665e-08, 3.654146194458e-08, 3.85564470291138e-08, 4.05360126495362e-08, 4.25753784179687e-08, 4.44810247421264e-08, 4.64640522003174e-08, 4.84134578704834e-08, 5.0360894203186e-08, 5.23087310791016e-08, 5.41706848144531e-08, 5.61122369766235e-08, 5.80254411697388e-08, 5.99296045303345e-08, 6.17995834350585e-08, 6.36650896072387e-08, 6.55740404129029e-08, 6.74563980102539e-08, 6.92941617965698e-08, 7.11823606491089e-08, 7.30168533325195e-08, 7.49124813079834e-08, 7.67757225036621e-08, 7.86007070541382e-08, 8.04677534103393e-08, 8.23359251022339e-08, 8.42034244537354e-08, 8.60402822494507e-08, 8.78436994552612e-08, 8.97126626968383e-08, 9.15588283538818e-08, 9.34039449691773e-08, 9.52537822723388e-08, 9.70710515975952e-08, 9.8919587135315e-08, 1.00779604911804e-07, 1.02571730613709e-07, 1.04448261260986e-07, 1.06267914772034e-07, 1.08109493255615e-07, 1.09986324310303e-07, 1.11741886138916e-07, 1.13620657920837e-07, 1.15449953079224e-07, 1.17288198471069e-07, 1.19147958755493e-07, 1.20904679298401e-07, 1.22782654762268e-07, 1.24627943038941e-07, 1.26412239074707e-07, 1.28273358345032e-07, 1.30083060264587e-07, 1.31924557685852e-07, 1.3378963470459e-07, 1.35558824539184e-07, 1.37415685653687e-07, 1.39248471260071e-07, 1.41111197471619e-07, 1.42928810119629e-07, 1.44692940711975e-07, 1.46567759513855e-07, 1.48380722999573e-07, 1.50204873085022e-07, 1.52055225372315e-07, 1.53859133720398e-07, 1.55690093040466e-07, 1.57527613639832e-07, 1.59333219528198e-07, 1.61180992126465e-07, 1.62985653877258e-07, 1.64833674430847e-07, 1.66662635803223e-07, 1.68453230857849e-07, 1.70259857177734e-07, 1.72122559547425e-07, 1.73938097953796e-07, 1.75762896537781e-07, 1.7755699634552e-07, 1.79424700736999e-07, 1.81225800514221e-07, 1.83002734184265e-07, 1.84867486953735e-07, 1.8625458240509e-07]}]
  in  "Subtract from 2T":cluster{dbl[], dbl[]}[](graph)=[{[-0.0489748717948718, -0.0484620512820513, -0.0479492307692308, -0.0474364102564103, -0.0469235897435897, -0.0464107692307692, -0.0458979487179487, -0.0453851282051282, -0.0448723076923077, -0.0443594871794872, -0.0438466666666667, -0.0433338461538462, -0.0428210256410256, -0.0423082051282051, -0.0417953846153846, -0.0412825641025641, -0.0407697435897436, -0.0402569230769231, -0.0397441025641026, -0.0392312820512821, -0.0387184615384615, -0.038205641025641, -0.0376928205128205, -0.03718, -0.0366671794871795, -0.036154358974359, -0.0356415384615385, -0.0351287179487179, -0.0346158974358974, -0.0341030769230769, -0.0335902564102564, -0.0330774358974359, -0.0325646153846154, -0.0320517948717949, -0.0315389743589744, -0.0310261538461539, -0.0305133333333333, -0.0300005128205128, -0.0294876923076923, -0.0289748717948718, -0.0284620512820513, -0.0279492307692308, -0.0274364102564103, -0.0269235897435897, -0.0264107692307692, -0.0258979487179487, -0.0253851282051282, -0.0248723076923077, -0.0243594871794872, -0.0238466666666667, -0.0233338461538462, -0.0228210256410256, -0.0223082051282051, -0.0217953846153846, -0.0212825641025641, -0.0207697435897436, -0.0202569230769231, -0.0197441025641026, -0.0192312820512821, -0.0187184615384615, -0.018205641025641, -0.0176928205128205, -0.01718, -0.0166671794871795, -0.016154358974359, -0.0156415384615385, -0.0151287179487179, -0.0146158974358974, -0.0141030769230769, -0.0135902564102564, -0.0130774358974359, -0.0125646153846154, -0.0120517948717949, -0.0115389743589744, -0.0110261538461539, -0.0105133333333333, -0.0100005128205128, -0.00948769230769232, -0.0089748717948718, -0.00846205128205129, -0.00794923076923078, -0.00743641025641026, -0.00692358974358975, -0.00641076923076923, -0.00589794871794873, -0.00538512820512821, -0.0048723076923077, -0.00435948717948719, -0.00384666666666667, -0.00333384615384616, -0.00282102564102565, -0.00230820512820513, -0.00179538461538462, -0.00128256410256411, -0.000769743589743595, -0.000256923076923082, 0.00025589743589743, 0.000768717948717944, 0.00128153846153846, 0.00179435897435897, 0.00230717948717948, 0.00282, 0.00333282051282051, 0.00384564102564102, 0.00435846153846153, 0.00487128205128205, 0.00538410256410256, 0.00589692307692307, 0.00640974358974358, 0.0069225641025641, 0.00743538461538461, 0.00794820512820512, 0.00846102564102563, 0.00897384615384614, 0.00948666666666666, 0.00999948717948717, 0.0105123076923077, 0.0110251282051282, 0.0115379487179487, 0.0120507692307692, 0.0125635897435897, 0.0130764102564102, 0.0135892307692308, 0.0141020512820513, 0.0146148717948718, 0.0151276923076923, 0.0156405128205128, 0.0161533333333333, 0.0166661538461538, 0.0171789743589743, 0.0176917948717949, 0.0182046153846154, 0.0187174358974359, 0.0192302564102564, 0.0197430769230769, 0.0202558974358974, 0.0207687179487179, 0.0212815384615385, 0.021794358974359, 0.0223071794871795, 0.02282, 0.0233328205128205, 0.023845641025641, 0.0243584615384615, 0.024871282051282, 0.0253841025641026, 0.0258969230769231, 0.0264097435897436, 0.0269225641025641, 0.0274353846153846, 0.0279482051282051, 0.0284610256410256, 0.0289738461538461, 0.0294866666666667, 0.0299994871794872, 0.0305123076923077, 0.0310251282051282, 0.0315379487179487, 0.0320507692307692, 0.0325635897435897, 0.0330764102564102, 0.0335892307692308, 0.0341020512820513, 0.0346148717948718, 0.0351276923076923, 0.0356405128205128, 0.0361533333333333, 0.0366661538461538, 0.0371789743589744, 0.0376917948717949, 0.0382046153846154, 0.0387174358974359, 0.0392302564102564, 0.0397430769230769, 0.0402558974358974, 0.0407687179487179, 0.0412815384615385, 0.041794358974359, 0.0423071794871795, 0.04282, 0.0433328205128205, 0.043845641025641, 0.0443584615384615, 0.044871282051282, 0.0453841025641026, 0.0458969230769231, 0.0464097435897436, 0.0469225641025641, 0.0474353846153846, 0.0479482051282051, 0.0484610256410256, 0.0489738461538461, 0.0494866666666667, 0.0498717948717949, 0.0494876923076923, 0.0489748717948718], [-1.65623290538788e-07, -1.64366676807403e-07, -1.6270928144455e-07, -1.60995314121246e-07, -1.59361979961395e-07, -1.57630341053009e-07, -1.55973608493805e-07, -1.54295709133148e-07, -1.52605640888214e-07, -1.50912983417511e-07, -1.49226620197296e-07, -1.475466132164e-07, -1.4587922334671e-07, -1.44224812984467e-07, -1.42522161006927e-07, -1.40824573040009e-07, -1.39135282039642e-07, -1.37492110729217e-07, -1.35790302753449e-07, -1.34116337299347e-07, -1.3245673418045e-07, -1.30749747753143e-07, -1.29089500904083e-07, -1.27423355579376e-07, -1.25717866420746e-07, -1.24082887172699e-07, -1.22372944355011e-07, -1.20709631443024e-07, -1.19034564495087e-07, -1.17329704761505e-07, -1.15688488483429e-07, -1.14004456996918e-07, -1.12311146259308e-07, -1.10657756328583e-07, -1.08971536159515e-07, -1.07327582836151e-07, -1.05632841587067e-07, -1.03951957225799e-07, -1.02282211780548e-07, -1.00602662563324e-07, -9.89398980140688e-08, -9.7249834537506e-08, -9.55907654762268e-08, -9.39223980903626e-08, -9.22377514839173e-08, -9.05766463279724e-08, -8.88806271553041e-08, -8.71998667716979e-08, -8.5557324886322e-08, -8.3875367641449e-08, -8.22046256065369e-08, -8.05323719978333e-08, -7.88461947441101e-08, -7.71867775917053e-08, -7.54862999916077e-08, -7.38244128227235e-08, -7.21955704689026e-08, -7.04725193977356e-08, -6.88083815574646e-08, -6.71566367149353e-08, -6.54385638237e-08, -6.38467431068419e-08, -6.2143075466156e-08, -6.04572749137879e-08, -5.87578082084656e-08, -5.70901560783387e-08, -5.54495358467102e-08, -5.37617182731628e-08, -5.20728945732117e-08, -5.04058623313903e-08, -4.87095475196839e-08, -4.7027313709259e-08, -4.53420376777649e-08, -4.36465048789978e-08, -4.19709610939026e-08, -4.02621626853943e-08, -3.85657000541687e-08, -3.68744158744812e-08, -3.51532435417175e-08, -3.34769129753113e-08, -3.17414307594299e-08, -3.00291275978088e-08, -2.82754874229431e-08, -2.65537762641907e-08, -2.48121857643128e-08, -2.30595564842224e-08, -2.12988495826721e-08, -1.95376849174499e-08, -1.77134680747986e-08, -1.59451270103455e-08, -1.41137337684631e-08, -1.22836995124817e-08, -1.0463182926178e-08, -8.59805345535279e-09, -6.7025065422058e-09, -4.80121850967407e-09, -2.85165071487427e-09, -9.28266048431397e-10, 1.10090494155884e-09, 3.14129114151001e-09, 5.0296664237976e-09, 7.03333139419556e-09, 8.91797304153442e-09, 1.08097529411316e-08, 1.2684600353241e-08, 1.44707369804382e-08, 1.63167977333069e-08, 1.8137309551239e-08, 1.99206042289734e-08, 2.17427086830139e-08, 2.34424328804016e-08, 2.52212119102478e-08, 2.69481062889099e-08, 2.87198233604431e-08, 3.04226469993591e-08, 3.21653485298157e-08, 3.38376879692077e-08, 3.55852150917053e-08, 3.72413992881775e-08, 3.89493918418884e-08, 4.06432223320008e-08, 4.23262333869934e-08, 4.40259337425232e-08, 4.56713366508484e-08, 4.73501849174499e-08, 4.90331721305847e-08, 5.07016587257386e-08, 5.23561406135559e-08, 5.40348935127259e-08, 5.56952404975891e-08, 5.73605847358704e-08, 5.9005024433136e-08, 6.06807923316955e-08, 6.23321557044983e-08, 6.40054345130921e-08, 6.56539988517761e-08, 6.72944521903992e-08, 6.89370369911194e-08, 7.06165385246277e-08, 7.22667288780212e-08, 7.39102435111999e-08, 7.55544304847718e-08, 7.72129702568054e-08, 7.88719964027404e-08, 8.05214047431947e-08, 8.21746850013733e-08, 8.3821895122528e-08, 8.54652380943299e-08, 8.71282458305359e-08, 8.87489199638366e-08, 9.04205203056335e-08, 9.2069251537323e-08, 9.37054467201232e-08, 9.53875327110291e-08, 9.69822192192079e-08, 9.86451411247254e-08, 1.00279037952423e-07, 1.0192996263504e-07, 1.03610188961029e-07, 1.05209062099457e-07, 1.06879980564117e-07, 1.08527138233185e-07, 1.1013329744339e-07, 1.11793959140778e-07, 1.13420279026032e-07, 1.15060799121857e-07, 1.16741449832916e-07, 1.18345229625702e-07, 1.19993097782135e-07, 1.21638219356537e-07, 1.23298089504242e-07, 1.24929182529449e-07, 1.26532180309296e-07, 1.28197796344757e-07, 1.29832246303558e-07, 1.31473739147186e-07, 1.33135645389557e-07, 1.34764506816864e-07, 1.36387865543365e-07, 1.38040716648102e-07, 1.39671413898468e-07, 1.41305329799652e-07, 1.42935883998871e-07, 1.445840716362e-07, 1.46223919391632e-07, 1.47864863872528e-07, 1.49482581615448e-07, 1.51141016483307e-07, 1.52767264842987e-07, 1.54417779445648e-07, 1.56036422252655e-07, 1.57684009075165e-07, 1.59307806491852e-07, 1.60909650325775e-07, 1.62571938037872e-07, 1.63812067508697e-07]}]
  in  "offset":i32=8
  in  "length":i32=1
  in  "stop":bool
  in  "decimate files":i32=1
  out "I vs V2T":cluster{dbl[], dbl[]}[](graph)=[{[-0.0489748717948718, -0.0484620512820513, -0.0479492307692308, -0.0474364102564103, -0.0469235897435897, -0.0464107692307692, -0.0458979487179487, -0.0453851282051282, -0.0448723076923077, -0.0443594871794872, -0.0438466666666667, -0.0433338461538462, -0.0428210256410256, -0.0423082051282051, -0.0417953846153846, -0.0412825641025641, -0.0407697435897436, -0.0402569230769231, -0.0397441025641026, -0.0392312820512821, -0.0387184615384615, -0.038205641025641, -0.0376928205128205, -0.03718, -0.0366671794871795, -0.036154358974359, -0.0356415384615385, -0.0351287179487179, -0.0346158974358974, -0.0341030769230769, -0.0335902564102564, -0.0330774358974359, -0.0325646153846154, -0.0320517948717949, -0.0315389743589744, -0.0310261538461539, -0.0305133333333333, -0.0300005128205128, -0.0294876923076923, -0.0289748717948718, -0.0284620512820513, -0.0279492307692308, -0.0274364102564103, -0.0269235897435897, -0.0264107692307692, -0.0258979487179487, -0.0253851282051282, -0.0248723076923077, -0.0243594871794872, -0.0238466666666667, -0.0233338461538462, -0.0228210256410256, -0.0223082051282051, -0.0217953846153846, -0.0212825641025641, -0.0207697435897436, -0.0202569230769231, -0.0197441025641026, -0.0192312820512821, -0.0187184615384615, -0.018205641025641, -0.0176928205128205, -0.01718, -0.0166671794871795, -0.016154358974359, -0.0156415384615385, -0.0151287179487179, -0.0146158974358974, -0.0141030769230769, -0.0135902564102564, -0.0130774358974359, -0.0125646153846154, -0.0120517948717949, -0.0115389743589744, -0.0110261538461539, -0.0105133333333333, -0.0100005128205128, -0.00948769230769232, -0.0089748717948718, -0.00846205128205129, -0.00794923076923078, -0.00743641025641026, -0.00692358974358975, -0.00641076923076923, -0.00589794871794873, -0.00538512820512821, -0.0048723076923077, -0.00435948717948719, -0.00384666666666667, -0.00333384615384616, -0.00282102564102565, -0.00230820512820513, -0.00179538461538462, -0.00128256410256411, -0.000769743589743595, -0.000256923076923082, 0.00025589743589743, 0.000768717948717944, 0.00128153846153846, 0.00179435897435897, 0.00230717948717948, 0.00282, 0.00333282051282051, 0.00384564102564102, 0.00435846153846153, 0.00487128205128205, 0.00538410256410256, 0.00589692307692307, 0.00640974358974358, 0.0069225641025641, 0.00743538461538461, 0.00794820512820512, 0.00846102564102563, 0.00897384615384614, 0.00948666666666666, 0.00999948717948717, 0.0105123076923077, 0.0110251282051282, 0.0115379487179487, 0.0120507692307692, 0.0125635897435897, 0.0130764102564102, 0.0135892307692308, 0.0141020512820513, 0.0146148717948718, 0.0151276923076923, 0.0156405128205128, 0.0161533333333333, 0.0166661538461538, 0.0171789743589743, 0.0176917948717949, 0.0182046153846154, 0.0187174358974359, 0.0192302564102564, 0.0197430769230769, 0.0202558974358974, 0.0207687179487179, 0.0212815384615385, 0.021794358974359, 0.0223071794871795, 0.02282, 0.0233328205128205, 0.023845641025641, 0.0243584615384615, 0.024871282051282, 0.0253841025641026, 0.0258969230769231, 0.0264097435897436, 0.0269225641025641, 0.0274353846153846, 0.0279482051282051, 0.0284610256410256, 0.0289738461538461, 0.0294866666666667, 0.0299994871794872, 0.0305123076923077, 0.0310251282051282, 0.0315379487179487, 0.0320507692307692, 0.0325635897435897, 0.0330764102564102, 0.0335892307692308, 0.0341020512820513, 0.0346148717948718, 0.0351276923076923, 0.0356405128205128, 0.0361533333333333, 0.0366661538461538, 0.0371789743589744, 0.0376917948717949, 0.0382046153846154, 0.0387174358974359, 0.0392302564102564, 0.0397430769230769, 0.0402558974358974, 0.0407687179487179, 0.0412815384615385, 0.041794358974359, 0.0423071794871795, 0.04282, 0.0433328205128205, 0.043845641025641, 0.0443584615384615, 0.044871282051282, 0.0453841025641026, 0.0458969230769231, 0.0464097435897436, 0.0469225641025641, 0.0474353846153846, 0.0479482051282051, 0.0484610256410256, 0.0489738461538461, 0.0494866666666667, 0.0498717948717949, 0.0494876923076923, 0.0489748717948718], [-1.88530516624451e-07, -1.87133288383484e-07, -1.85253167152405e-07, -1.83320441246033e-07, -1.81518726348877e-07, -1.79542255401611e-07, -1.77687950134277e-07, -1.75797801017761e-07, -1.73898572921753e-07, -1.71995229721069e-07, -1.70092630386353e-07, -1.68203616142273e-07, -1.6635901927948e-07, -1.64455137252808e-07, -1.62550988197327e-07, -1.60638189315796e-07, -1.58735628128052e-07, -1.56911063194275e-07, -1.54978852272034e-07, -1.53096804618836e-07, -1.51216950416565e-07, -1.49291834831238e-07, -1.47456007003784e-07, -1.45557689666748e-07, -1.4364326953888e-07, -1.41811571121216e-07, -1.3987343788147e-07, -1.38007555007935e-07, -1.36112055778503e-07, -1.34210629463196e-07, -1.3238597869873e-07, -1.30467686653137e-07, -1.28578906059265e-07, -1.26701898574829e-07, -1.24821209907532e-07, -1.22998299598694e-07, -1.21071562767029e-07, -1.19200682640076e-07, -1.17325396537781e-07, -1.15441784858704e-07, -1.1358193397522e-07, -1.11678218841553e-07, -1.09816336631775e-07, -1.0796443939209e-07, -1.06044731140137e-07, -1.04197044372559e-07, -1.02285056114197e-07, -1.00400342941284e-07, -9.85824632644653e-08, -9.66873502731323e-08, -9.47991418838502e-08, -9.29165840148925e-08, -9.10269689559937e-08, -8.91835737228393e-08, -8.72648000717163e-08, -8.53948640823364e-08, -8.35837936401368e-08, -8.16421175003052e-08, -7.9793062210083e-08, -7.79200601577759e-08, -7.59902238845825e-08, -7.42254400253296e-08, -7.22940492630005e-08, -7.04062414169312e-08, -6.84745645523071e-08, -6.65928602218628e-08, -6.47673559188843e-08, -6.28309917449951e-08, -6.0914454460144e-08, -5.90352773666382e-08, -5.7114372253418e-08, -5.52046394348144e-08, -5.32772445678711e-08, -5.13371229171753e-08, -4.94526720046997e-08, -4.74649143218994e-08, -4.55275678634644e-08, -4.35710477828979e-08, -4.159517288208e-08, -3.96825170516968e-08, -3.76472520828247e-08, -3.56490802764893e-08, -3.36032581329346e-08, -3.15900993347168e-08, -2.95552396774292e-08, -2.74624919891357e-08, -2.53818082809448e-08, -2.33121252059936e-08, -2.11334800720215e-08, -1.90311288833618e-08, -1.68199777603149e-08, -1.46402263641357e-08, -1.24739789962768e-08, -1.02206993103027e-08, -7.93179988861084e-09, -5.64008235931397e-09, -3.30891609191894e-09, -1.04283332824707e-09, 1.40513420104981e-09, 3.84415149688721e-09, 6.134033203125e-09, 8.53836059570313e-09, 1.08101654052734e-08, 1.31109428405762e-08, 1.53783369064331e-08, 1.75216150283813e-08, 1.97556734085083e-08, 2.19318246841431e-08, 2.40856266021728e-08, 2.62651681900024e-08, 2.82614612579346e-08, 3.04032325744629e-08, 3.24541425704956e-08, 3.45364236831665e-08, 3.654146194458e-08, 3.85564470291138e-08, 4.05360126495362e-08, 4.25753784179687e-08, 4.44810247421264e-08, 4.64640522003174e-08, 4.84134578704834e-08, 5.0360894203186e-08, 5.23087310791016e-08, 5.41706848144531e-08, 5.61122369766235e-08, 5.80254411697388e-08, 5.99296045303345e-08, 6.17995834350585e-08, 6.36650896072387e-08, 6.55740404129029e-08, 6.74563980102539e-08, 6.92941617965698e-08, 7.11823606491089e-08, 7.30168533325195e-08, 7.49124813079834e-08, 7.67757225036621e-08, 7.86007070541382e-08, 8.04677534103393e-08, 8.23359251022339e-08, 8.42034244537354e-08, 8.60402822494507e-08, 8.78436994552612e-08, 8.97126626968383e-08, 9.15588283538818e-08, 9.34039449691773e-08, 9.52537822723388e-08, 9.70710515975952e-08, 9.8919587135315e-08, 1.00779604911804e-07, 1.02571730613709e-07, 1.04448261260986e-07, 1.06267914772034e-07, 1.08109493255615e-07, 1.09986324310303e-07, 1.11741886138916e-07, 1.13620657920837e-07, 1.15449953079224e-07, 1.17288198471069e-07, 1.19147958755493e-07, 1.20904679298401e-07, 1.22782654762268e-07, 1.24627943038941e-07, 1.26412239074707e-07, 1.28273358345032e-07, 1.30083060264587e-07, 1.31924557685852e-07, 1.3378963470459e-07, 1.35558824539184e-07, 1.37415685653687e-07, 1.39248471260071e-07, 1.41111197471619e-07, 1.42928810119629e-07, 1.44692940711975e-07, 1.46567759513855e-07, 1.48380722999573e-07, 1.50204873085022e-07, 1.52055225372315e-07, 1.53859133720398e-07, 1.55690093040466e-07, 1.57527613639832e-07, 1.59333219528198e-07, 1.61180992126465e-07, 1.62985653877258e-07, 1.64833674430847e-07, 1.66662635803223e-07, 1.68453230857849e-07, 1.70259857177734e-07, 1.72122559547425e-07, 1.73938097953796e-07, 1.75762896537781e-07, 1.7755699634552e-07, 1.79424700736999e-07, 1.81225800514221e-07, 1.83002734184265e-07, 1.84867486953735e-07, 1.8625458240509e-07]}]
  out "Subtracted \nI vs V4T":cluster{dbl[], dbl[]}[](graph)=[{[-0.020298805594444295, -0.020143332123756498, -0.019935172677040203, -0.019711892008781505, -0.019499069094658004, -0.019296326518058897, -0.0190861269235612, -0.018870721936226, -0.0186526147127153, -0.0184441012144091, -0.018240182995796404, -0.018026167988777403, -0.017805154204368796, -0.0175968400239946, -0.017388032078743197, -0.017181379437446798, -0.016960291981697302, -0.016742527604103302, -0.0165384343862536, -0.0163279012441638, -0.0161165035963061, -0.0158924008607867, -0.0156821869611742, -0.015477146983146901, -0.015263935208320902, -0.0150432082414629, -0.014828914046287701, -0.0146212004423143, -0.0144141832590105, -0.0141964107751848, -0.0139734686613085, -0.013768090128898802, -0.0135563558340074, -0.013346166729927202, -0.013120899081230299, -0.0129057987928392, -0.012701104283332999, -0.012487238287925912, -0.01226870453357717, -0.01204702484607715, -0.01183656013011947, -0.01162859666347524, -0.01141238462924974, -0.01118832433223746, -0.010975580811500699, -0.01076415216922773, -0.010553850293159662, -0.010330365061760138, -0.010109158396721092, -0.009902112841606301, -0.00968768084049235, -0.00947194325923932, -0.009244939923286621, -0.009032684683799868, -0.00882454001903547, -0.00860845100879677, -0.00838605582714088, -0.008168872952461409, -0.00795692384243022, -0.007747506260871981, -0.007525480151176509, -0.007301862120628491, -0.007093491911888181, -0.0068792678117752595, -0.0066681920289994095, -0.00644138252735143, -0.0062280436754227, -0.00602158486843118, -0.005808955550193789, -0.00559199845790865, -0.00537080562114718, -0.005163264632225051, -0.0049578579664230306, -0.00474451506137847, -0.004523096442222571, -0.004317351222038229, -0.0041118384599685195, -0.0039091233015059994, -0.00369388210773464, -0.0034842001199722, -0.0032883435487746897, -0.0030877457857131797, -0.0028865646123886, -0.0026763523817062403, -0.00248287928104402, -0.0022957037687301902, -0.0021012431383133304, -0.0018998574018478898, -0.00170761549472813, -0.0015246480703354297, -0.0013457845449447899, -0.0011569598913192998, -0.0009671784639358609, -0.000797939419746412, -0.0006248732805252139, -0.00045578753948211396, -0.00027331769466399497, -0.00010534942150116299, 4.9853920936584e-05, 0.00021248924732208502, 0.00038257944583893004, 0.000559727311134333, 0.000726794123649592, 0.000892312169075, 0.00107245266437529, 0.0012648783922195202, 0.00144211494922634, 0.00162198793888088, 0.0018035722970962, 0.00200244796276088, 0.0021988219022750504, 0.0023840004205703496, 0.00257733285427093, 0.0027730993032455404, 0.00298340857028962, 0.00318200647830965, 0.0033764384984970304, 0.00358172023296359, 0.0037975507974625003, 0.00400608170032506, 0.004211035609245349, 0.00441424405574801, 0.00463290369510651, 0.004853630900382989, 0.00505880463123321, 0.00527102982997892, 0.00548183524608609, 0.00570913612842555, 0.0059262028932570805, 0.0061337746381759, 0.006350606799125561, 0.00657308328151695, 0.006797502160072209, 0.00701170980930318, 0.007223751902580171, 0.007445839762687629, 0.0076745249032973495, 0.00788892495632163, 0.008105991482734609, 0.00832066643238058, 0.00854929745197286, 0.008773327469825608, 0.008985962748527383, 0.009204881548881421, 0.00942662870883931, 0.009656422495841838, 0.009873687624931172, 0.01008750140666952, 0.010308032870292512, 0.010535851359367219, 0.010755051493644521, 0.01097254836559275, 0.011186535954475272, 0.01141592419147475, 0.01164573872089373, 0.01185890591144548, 0.01207890450954417, 0.01229698598384842, 0.0125287271738051, 0.012748497128486448, 0.012961129307746701, 0.0131815141439436, 0.0134082280397413, 0.013634177565574501, 0.0138529192209242, 0.014067153573036, 0.014290386795997399, 0.0145212532281873, 0.0147375079393385, 0.014956275105476199, 0.015173210740089201, 0.0154038113355635, 0.0156266974210737, 0.0158396693468092, 0.016059869408607298, 0.0162831009626387, 0.0165129681825636, 0.0167303055524824, 0.016944220423698197, 0.0171680797338483, 0.0173991161584852, 0.017618041872978, 0.017834319472312697, 0.018048580527305402, 0.0182773231267927, 0.018506924033164802, 0.0187209612131117, 0.018940549969673003, 0.0191605340242385, 0.019393757939338598, 0.019613784909248304, 0.0198268069028853, 0.0200480521917343, 0.020275678992271395, 0.0205016232728957, 0.0206638196706772], [0.0, 0.0, 0.0, 0.0, 0.0, 0.0, 0.0, 0.0, 0.0, 0.0, 0.0, 0.0, 0.0, 0.0, 0.0, 0.0, 0.0, 0.0, 0.0, 0.0, 0.0, 0.0, 0.0, 0.0, 0.0, 0.0, 0.0, 0.0, 0.0, 0.0, 0.0, 0.0, 0.0, 0.0, 0.0, 0.0, 0.0, 0.0, 0.0, 0.0, 0.0, 0.0, 0.0, 0.0, 0.0, 0.0, 0.0, 0.0, 0.0, 0.0, 0.0, 0.0, 0.0, 0.0, 0.0, 0.0, 0.0, 0.0, 0.0, 0.0, 0.0, 0.0, 0.0, 0.0, 0.0, 0.0, 0.0, 0.0, 0.0, 0.0, 0.0, 0.0, 0.0, 0.0, 0.0, 0.0, 0.0, 0.0, 0.0, 0.0, 0.0, 0.0, 0.0, 0.0, 0.0, 0.0, 0.0, 0.0, 0.0, 0.0, 0.0, 0.0, 0.0, 0.0, 0.0, 0.0, 0.0, 0.0, 0.0, 0.0, 0.0, 0.0, 0.0, 0.0, 0.0, 0.0, 0.0, 0.0, 0.0, 0.0, 0.0, 0.0, 0.0, 0.0, 0.0, 0.0, 0.0, 0.0, 0.0, 0.0, 0.0, 0.0, 0.0, 0.0, 0.0, 0.0, 0.0, 0.0, 0.0, 0.0, 0.0, 0.0, 0.0, 0.0, 0.0, 0.0, 0.0, 0.0, 0.0, 0.0, 0.0, 0.0, 0.0, 0.0, 0.0, 0.0, 0.0, 0.0, 0.0, 0.0, 0.0, 0.0, 0.0, 0.0, 0.0, 0.0, 0.0, 0.0, 0.0, 0.0, 0.0, 0.0, 0.0, 0.0, 0.0, 0.0, 0.0, 0.0, 0.0, 0.0, 0.0, 0.0, 0.0, 0.0, 0.0, 0.0, 0.0, 0.0, 0.0, 0.0, 0.0, 0.0, 0.0, 0.0, 0.0, 0.0, 0.0, 0.0, 0.0, 0.0, 0.0, 0.0, 0.0, 0.0, 0.0, 0.0]}]
  out "Vslow":dbl=0.99993349609375
  out "Vfast":dbl=0.099648
  out "I vs V4T":cluster{dbl[], dbl[]}[](graph)=[{[-0.020298805594444295, -0.020143332123756498, -0.019935172677040203, -0.019711892008781505, -0.019499069094658004, -0.019296326518058897, -0.0190861269235612, -0.018870721936226, -0.0186526147127153, -0.0184441012144091, -0.018240182995796404, -0.018026167988777403, -0.017805154204368796, -0.0175968400239946, -0.017388032078743197, -0.017181379437446798, -0.016960291981697302, -0.016742527604103302, -0.0165384343862536, -0.0163279012441638, -0.0161165035963061, -0.0158924008607867, -0.0156821869611742, -0.015477146983146901, -0.015263935208320902, -0.0150432082414629, -0.014828914046287701, -0.0146212004423143, -0.0144141832590105, -0.0141964107751848, -0.0139734686613085, -0.013768090128898802, -0.0135563558340074, -0.013346166729927202, -0.013120899081230299, -0.0129057987928392, -0.012701104283332999, -0.012487238287925912, -0.01226870453357717, -0.01204702484607715, -0.01183656013011947, -0.01162859666347524, -0.01141238462924974, -0.01118832433223746, -0.010975580811500699, -0.01076415216922773, -0.010553850293159662, -0.010330365061760138, -0.010109158396721092, -0.009902112841606301, -0.00968768084049235, -0.00947194325923932, -0.009244939923286621, -0.009032684683799868, -0.00882454001903547, -0.00860845100879677, -0.00838605582714088, -0.008168872952461409, -0.00795692384243022, -0.007747506260871981, -0.007525480151176509, -0.007301862120628491, -0.007093491911888181, -0.0068792678117752595, -0.0066681920289994095, -0.00644138252735143, -0.0062280436754227, -0.00602158486843118, -0.005808955550193789, -0.00559199845790865, -0.00537080562114718, -0.005163264632225051, -0.0049578579664230306, -0.00474451506137847, -0.004523096442222571, -0.004317351222038229, -0.0041118384599685195, -0.0039091233015059994, -0.00369388210773464, -0.0034842001199722, -0.0032883435487746897, -0.0030877457857131797, -0.0028865646123886, -0.0026763523817062403, -0.00248287928104402, -0.0022957037687301902, -0.0021012431383133304, -0.0018998574018478898, -0.00170761549472813, -0.0015246480703354297, -0.0013457845449447899, -0.0011569598913192998, -0.0009671784639358609, -0.000797939419746412, -0.0006248732805252139, -0.00045578753948211396, -0.00027331769466399497, -0.00010534942150116299, 4.9853920936584e-05, 0.00021248924732208502, 0.00038257944583893004, 0.000559727311134333, 0.000726794123649592, 0.000892312169075, 0.00107245266437529, 0.0012648783922195202, 0.00144211494922634, 0.00162198793888088, 0.0018035722970962, 0.00200244796276088, 0.0021988219022750504, 0.0023840004205703496, 0.00257733285427093, 0.0027730993032455404, 0.00298340857028962, 0.00318200647830965, 0.0033764384984970304, 0.00358172023296359, 0.0037975507974625003, 0.00400608170032506, 0.004211035609245349, 0.00441424405574801, 0.00463290369510651, 0.004853630900382989, 0.00505880463123321, 0.00527102982997892, 0.00548183524608609, 0.00570913612842555, 0.0059262028932570805, 0.0061337746381759, 0.006350606799125561, 0.00657308328151695, 0.006797502160072209, 0.00701170980930318, 0.007223751902580171, 0.007445839762687629, 0.0076745249032973495, 0.00788892495632163, 0.008105991482734609, 0.00832066643238058, 0.00854929745197286, 0.008773327469825608, 0.008985962748527383, 0.009204881548881421, 0.00942662870883931, 0.009656422495841838, 0.009873687624931172, 0.01008750140666952, 0.010308032870292512, 0.010535851359367219, 0.010755051493644521, 0.01097254836559275, 0.011186535954475272, 0.01141592419147475, 0.01164573872089373, 0.01185890591144548, 0.01207890450954417, 0.01229698598384842, 0.0125287271738051, 0.012748497128486448, 0.012961129307746701, 0.0131815141439436, 0.0134082280397413, 0.013634177565574501, 0.0138529192209242, 0.014067153573036, 0.014290386795997399, 0.0145212532281873, 0.0147375079393385, 0.014956275105476199, 0.015173210740089201, 0.0154038113355635, 0.0156266974210737, 0.0158396693468092, 0.016059869408607298, 0.0162831009626387, 0.0165129681825636, 0.0167303055524824, 0.016944220423698197, 0.0171680797338483, 0.0173991161584852, 0.017618041872978, 0.017834319472312697, 0.018048580527305402, 0.0182773231267927, 0.018506924033164802, 0.0187209612131117, 0.018940549969673003, 0.0191605340242385, 0.019393757939338598, 0.019613784909248304, 0.0198268069028853, 0.0200480521917343, 0.020275678992271395, 0.0205016232728957, 0.0206638196706772], [-1.88530516624451e-07, -1.87133288383484e-07, -1.85253167152405e-07, -1.83320441246033e-07, -1.81518726348877e-07, -1.79542255401611e-07, -1.77687950134277e-07, -1.75797801017761e-07, -1.73898572921753e-07, -1.71995229721069e-07, -1.70092630386353e-07, -1.68203616142273e-07, -1.6635901927948e-07, -1.64455137252808e-07, -1.62550988197327e-07, -1.60638189315796e-07, -1.58735628128052e-07, -1.56911063194275e-07, -1.54978852272034e-07, -1.53096804618836e-07, -1.51216950416565e-07, -1.49291834831238e-07, -1.47456007003784e-07, -1.45557689666748e-07, -1.4364326953888e-07, -1.41811571121216e-07, -1.3987343788147e-07, -1.38007555007935e-07, -1.36112055778503e-07, -1.34210629463196e-07, -1.3238597869873e-07, -1.30467686653137e-07, -1.28578906059265e-07, -1.26701898574829e-07, -1.24821209907532e-07, -1.22998299598694e-07, -1.21071562767029e-07, -1.19200682640076e-07, -1.17325396537781e-07, -1.15441784858704e-07, -1.1358193397522e-07, -1.11678218841553e-07, -1.09816336631775e-07, -1.0796443939209e-07, -1.06044731140137e-07, -1.04197044372559e-07, -1.02285056114197e-07, -1.00400342941284e-07, -9.85824632644653e-08, -9.66873502731323e-08, -9.47991418838502e-08, -9.29165840148925e-08, -9.10269689559937e-08, -8.91835737228393e-08, -8.72648000717163e-08, -8.53948640823364e-08, -8.35837936401368e-08, -8.16421175003052e-08, -7.9793062210083e-08, -7.79200601577759e-08, -7.59902238845825e-08, -7.42254400253296e-08, -7.22940492630005e-08, -7.04062414169312e-08, -6.84745645523071e-08, -6.65928602218628e-08, -6.47673559188843e-08, -6.28309917449951e-08, -6.0914454460144e-08, -5.90352773666382e-08, -5.7114372253418e-08, -5.52046394348144e-08, -5.32772445678711e-08, -5.13371229171753e-08, -4.94526720046997e-08, -4.74649143218994e-08, -4.55275678634644e-08, -4.35710477828979e-08, -4.159517288208e-08, -3.96825170516968e-08, -3.76472520828247e-08, -3.56490802764893e-08, -3.36032581329346e-08, -3.15900993347168e-08, -2.95552396774292e-08, -2.74624919891357e-08, -2.53818082809448e-08, -2.33121252059936e-08, -2.11334800720215e-08, -1.90311288833618e-08, -1.68199777603149e-08, -1.46402263641357e-08, -1.24739789962768e-08, -1.02206993103027e-08, -7.93179988861084e-09, -5.64008235931397e-09, -3.30891609191894e-09, -1.04283332824707e-09, 1.40513420104981e-09, 3.84415149688721e-09, 6.134033203125e-09, 8.53836059570313e-09, 1.08101654052734e-08, 1.31109428405762e-08, 1.53783369064331e-08, 1.75216150283813e-08, 1.97556734085083e-08, 2.19318246841431e-08, 2.40856266021728e-08, 2.62651681900024e-08, 2.82614612579346e-08, 3.04032325744629e-08, 3.24541425704956e-08, 3.45364236831665e-08, 3.654146194458e-08, 3.85564470291138e-08, 4.05360126495362e-08, 4.25753784179687e-08, 4.44810247421264e-08, 4.64640522003174e-08, 4.84134578704834e-08, 5.0360894203186e-08, 5.23087310791016e-08, 5.41706848144531e-08, 5.61122369766235e-08, 5.80254411697388e-08, 5.99296045303345e-08, 6.17995834350585e-08, 6.36650896072387e-08, 6.55740404129029e-08, 6.74563980102539e-08, 6.92941617965698e-08, 7.11823606491089e-08, 7.30168533325195e-08, 7.49124813079834e-08, 7.67757225036621e-08, 7.86007070541382e-08, 8.04677534103393e-08, 8.23359251022339e-08, 8.42034244537354e-08, 8.60402822494507e-08, 8.78436994552612e-08, 8.97126626968383e-08, 9.15588283538818e-08, 9.34039449691773e-08, 9.52537822723388e-08, 9.70710515975952e-08, 9.8919587135315e-08, 1.00779604911804e-07, 1.02571730613709e-07, 1.04448261260986e-07, 1.06267914772034e-07, 1.08109493255615e-07, 1.09986324310303e-07, 1.11741886138916e-07, 1.13620657920837e-07, 1.15449953079224e-07, 1.17288198471069e-07, 1.19147958755493e-07, 1.20904679298401e-07, 1.22782654762268e-07, 1.24627943038941e-07, 1.26412239074707e-07, 1.28273358345032e-07, 1.30083060264587e-07, 1.31924557685852e-07, 1.3378963470459e-07, 1.35558824539184e-07, 1.37415685653687e-07, 1.39248471260071e-07, 1.41111197471619e-07, 1.42928810119629e-07, 1.44692940711975e-07, 1.46567759513855e-07, 1.48380722999573e-07, 1.50204873085022e-07, 1.52055225372315e-07, 1.53859133720398e-07, 1.55690093040466e-07, 1.57527613639832e-07, 1.59333219528198e-07, 1.61180992126465e-07, 1.62985653877258e-07, 1.64833674430847e-07, 1.66662635803223e-07, 1.68453230857849e-07, 1.70259857177734e-07, 1.72122559547425e-07, 1.73938097953796e-07, 1.75762896537781e-07, 1.7755699634552e-07, 1.79424700736999e-07, 1.81225800514221e-07, 1.83002734184265e-07, 1.84867486953735e-07, 1.8625458240509e-07]}]
  out "Subtracted\nI vs V2T":cluster{dbl[], dbl[]}[](graph)=[{[-0.0489748717948718, -0.0484620512820513, -0.0479492307692308, -0.0474364102564103, -0.0469235897435897, -0.0464107692307692, -0.0458979487179487, -0.0453851282051282, -0.0448723076923077, -0.0443594871794872, -0.0438466666666667, -0.0433338461538462, -0.0428210256410256, -0.0423082051282051, -0.0417953846153846, -0.0412825641025641, -0.0407697435897436, -0.0402569230769231, -0.0397441025641026, -0.0392312820512821, -0.0387184615384615, -0.038205641025641, -0.0376928205128205, -0.03718, -0.0366671794871795, -0.036154358974359, -0.0356415384615385, -0.0351287179487179, -0.0346158974358974, -0.0341030769230769, -0.0335902564102564, -0.0330774358974359, -0.0325646153846154, -0.0320517948717949, -0.0315389743589744, -0.0310261538461539, -0.0305133333333333, -0.0300005128205128, -0.0294876923076923, -0.0289748717948718, -0.0284620512820513, -0.0279492307692308, -0.0274364102564103, -0.0269235897435897, -0.0264107692307692, -0.0258979487179487, -0.0253851282051282, -0.0248723076923077, -0.0243594871794872, -0.0238466666666667, -0.0233338461538462, -0.0228210256410256, -0.0223082051282051, -0.0217953846153846, -0.0212825641025641, -0.0207697435897436, -0.0202569230769231, -0.0197441025641026, -0.0192312820512821, -0.0187184615384615, -0.018205641025641, -0.0176928205128205, -0.01718, -0.0166671794871795, -0.016154358974359, -0.0156415384615385, -0.0151287179487179, -0.0146158974358974, -0.0141030769230769, -0.0135902564102564, -0.0130774358974359, -0.0125646153846154, -0.0120517948717949, -0.0115389743589744, -0.0110261538461539, -0.0105133333333333, -0.0100005128205128, -0.00948769230769232, -0.0089748717948718, -0.00846205128205129, -0.00794923076923078, -0.00743641025641026, -0.00692358974358975, -0.00641076923076923, -0.00589794871794873, -0.00538512820512821, -0.0048723076923077, -0.00435948717948719, -0.00384666666666667, -0.00333384615384616, -0.00282102564102565, -0.00230820512820513, -0.00179538461538462, -0.00128256410256411, -0.000769743589743595, -0.000256923076923082, 0.00025589743589743, 0.000768717948717944, 0.00128153846153846, 0.00179435897435897, 0.00230717948717948, 0.00282, 0.00333282051282051, 0.00384564102564102, 0.00435846153846153, 0.00487128205128205, 0.00538410256410256, 0.00589692307692307, 0.00640974358974358, 0.0069225641025641, 0.00743538461538461, 0.00794820512820512, 0.00846102564102563, 0.00897384615384614, 0.00948666666666666, 0.00999948717948717, 0.0105123076923077, 0.0110251282051282, 0.0115379487179487, 0.0120507692307692, 0.0125635897435897, 0.0130764102564102, 0.0135892307692308, 0.0141020512820513, 0.0146148717948718, 0.0151276923076923, 0.0156405128205128, 0.0161533333333333, 0.0166661538461538, 0.0171789743589743, 0.0176917948717949, 0.0182046153846154, 0.0187174358974359, 0.0192302564102564, 0.0197430769230769, 0.0202558974358974, 0.0207687179487179, 0.0212815384615385, 0.021794358974359, 0.0223071794871795, 0.02282, 0.0233328205128205, 0.023845641025641, 0.0243584615384615, 0.024871282051282, 0.0253841025641026, 0.0258969230769231, 0.0264097435897436, 0.0269225641025641, 0.0274353846153846, 0.0279482051282051, 0.0284610256410256, 0.0289738461538461, 0.0294866666666667, 0.0299994871794872, 0.0305123076923077, 0.0310251282051282, 0.0315379487179487, 0.0320507692307692, 0.0325635897435897, 0.0330764102564102, 0.0335892307692308, 0.0341020512820513, 0.0346148717948718, 0.0351276923076923, 0.0356405128205128, 0.0361533333333333, 0.0366661538461538, 0.0371789743589744, 0.0376917948717949, 0.0382046153846154, 0.0387174358974359, 0.0392302564102564, 0.0397430769230769, 0.0402558974358974, 0.0407687179487179, 0.0412815384615385, 0.041794358974359, 0.0423071794871795, 0.04282, 0.0433328205128205, 0.043845641025641, 0.0443584615384615, 0.044871282051282, 0.0453841025641026, 0.0458969230769231, 0.0464097435897436, 0.0469225641025641, 0.0474353846153846, 0.0479482051282051, 0.0484610256410256, 0.0489738461538461, 0.0494866666666667, 0.0498717948717949, 0.0494876923076923, 0.0489748717948718], [-2.2907226085663017e-08, -2.2766611576081004e-08, -2.2543885707855005e-08, -2.232512712478698e-08, -2.2156746387482007e-08, -2.191191434860199e-08, -2.1714341640471997e-08, -2.150209188461301e-08, -2.1292932033539006e-08, -2.1082246303557996e-08, -2.0866010189056992e-08, -2.0657002925873005e-08, -2.047979593277e-08, -2.023032426834099e-08, -2.0028827190400018e-08, -1.9813616275786997e-08, -1.9600346088410018e-08, -1.941895246505802e-08, -1.9188549518584996e-08, -1.8980467319489024e-08, -1.876021623611502e-08, -1.8542087078094988e-08, -1.8366506099700995e-08, -1.8134334087371994e-08, -1.792540311813402e-08, -1.7728683948516998e-08, -1.7500493526458988e-08, -1.7297923564911008e-08, -1.707749128341599e-08, -1.6880924701691007e-08, -1.6697490215301003e-08, -1.6463229656218993e-08, -1.6267759799956997e-08, -1.6044142246245997e-08, -1.584967374801701e-08, -1.567071676254301e-08, -1.5438721179962e-08, -1.5248725414277e-08, -1.5043184757233006e-08, -1.483912229538e-08, -1.4642035961151196e-08, -1.4428384304046995e-08, -1.4225571155548207e-08, -1.4042041301727394e-08, -1.3806979656219707e-08, -1.3620398044586597e-08, -1.3404428958892909e-08, -1.3200476169586113e-08, -1.3025138378143298e-08, -1.28119826316833e-08, -1.2594516277313299e-08, -1.2384212017059206e-08, -1.2180774211883607e-08, -1.1996796131134e-08, -1.1778500080108606e-08, -1.1570451259612897e-08, -1.1388223171234206e-08, -1.11695981025696e-08, -1.0984680652618391e-08, -1.0763423442840605e-08, -1.055166006088249e-08, -1.0378696918487706e-08, -1.0150973796844502e-08, -9.948966503143302e-09, -9.716756343841493e-09, -9.502704143524096e-09, -9.317820072174096e-09, -9.069273471832303e-09, -8.841559886932298e-09, -8.6294150352479e-09, -8.404824733734103e-09, -8.177325725555402e-09, -7.935206890106198e-09, -7.690618038177499e-09, -7.481710910797098e-09, -7.202751636505104e-09, -6.9618678092956975e-09, -6.696631908416699e-09, -6.441929340362501e-09, -6.2056040763855e-09, -5.905821323394803e-09, -5.619952678680495e-09, -5.327770709991496e-09, -5.036323070526097e-09, -4.743053913116402e-09, -4.402935504913301e-09, -4.082958698272701e-09, -3.774440288543698e-09, -3.4200119972229006e-09, -3.0860018730163006e-09, -2.706243991851799e-09, -2.3565268516540003e-09, -2.0107960700988007e-09, -1.6226458549499095e-09, -1.2292933464050398e-09, -8.388638496399007e-10, -4.572653770446699e-10, -1.1456727981567307e-10, 3.042292594909701e-10, 7.028603553772e-10, 1.1043667793274005e-09, 1.50502920150757e-09, 1.892192363738981e-09, 2.301189899444599e-09, 2.6937365531921003e-09, 3.0508780479431e-09, 3.4388756752014e-09, 3.794515132904098e-09, 4.1650223731993995e-09, 4.5224595069885e-09, 4.819028377533001e-09, 5.182020664215099e-09, 5.506036281585702e-09, 5.816600322723401e-09, 6.118814945220904e-09, 6.391098499298095e-09, 6.698324680328501e-09, 6.9901633262634005e-09, 7.239625453948905e-09, 7.514660358428995e-09, 7.770235538482603e-09, 8.0346608161926e-09, 8.282797336578402e-09, 8.499348163604706e-09, 8.762052059173595e-09, 8.9922690391541e-09, 9.227945804595902e-09, 9.443442821502596e-09, 9.6301960945128e-09, 9.8787999153138e-09, 1.0095813274383495e-08, 1.0289137363433794e-08, 1.0501568317413413e-08, 1.0684697628021202e-08, 1.0907046794891307e-08, 1.1121723651886006e-08, 1.1306254863739008e-08, 1.15307164192199e-08, 1.171938657760619e-08, 1.19366955757142e-08, 1.2130038738250804e-08, 1.2289268970489393e-08, 1.2499692440032909e-08, 1.2686831951141405e-08, 1.2882540225982603e-08, 1.3079097270965511e-08, 1.3249156475067202e-08, 1.3454349040985097e-08, 1.36513590812681e-08, 1.38228106498724e-08, 1.4027740955352495e-08, 1.4198663234711005e-08, 1.4404046535491803e-08, 1.4598791599273898e-08, 1.4759666919708097e-08, 1.4975516796111595e-08, 1.5170915126800998e-08, 1.5358235836029e-08, 1.553776979446399e-08, 1.5695617198944002e-08, 1.5902674198150986e-08, 1.6100804805755996e-08, 1.627894163131701e-08, 1.647939920425399e-08, 1.6662781238554992e-08, 1.686375856399499e-08, 1.7048184871673983e-08, 1.7213594913482014e-08, 1.7422587871552004e-08, 1.761025190353401e-08, 1.7813107967377e-08, 1.799962759018e-08, 1.8160760402679016e-08, 1.8369963169098e-08, 1.8548476696014988e-08, 1.873113393783598e-08, 1.891957998275798e-08, 1.909462690353401e-08, 1.9302227497101004e-08, 1.9486896991729985e-08, 1.966180562973002e-08, 1.9875662326813002e-08, 2.0049769878387017e-08, 2.0249602794647002e-08, 2.0438716411590982e-08, 2.0588366985321005e-08, 2.0777275562286007e-08, 2.0981543064118017e-08, 2.117083311080901e-08, 2.1345117092133002e-08, 2.1520574092865e-08, 2.174069166183401e-08, 2.1917994022369005e-08, 2.2093083858490016e-08, 2.2295548915863008e-08, 2.2442514896392993e-08]}]
  in  "File or Folder Path":path=path "G:/.shortcut-targets-by-id/0B8-gGFa6hkR4XzJJMDlqZXVKRk0/ansom/Data/PPMS 3/SA40511C.20250205/08-IVWire1nd2_heating"
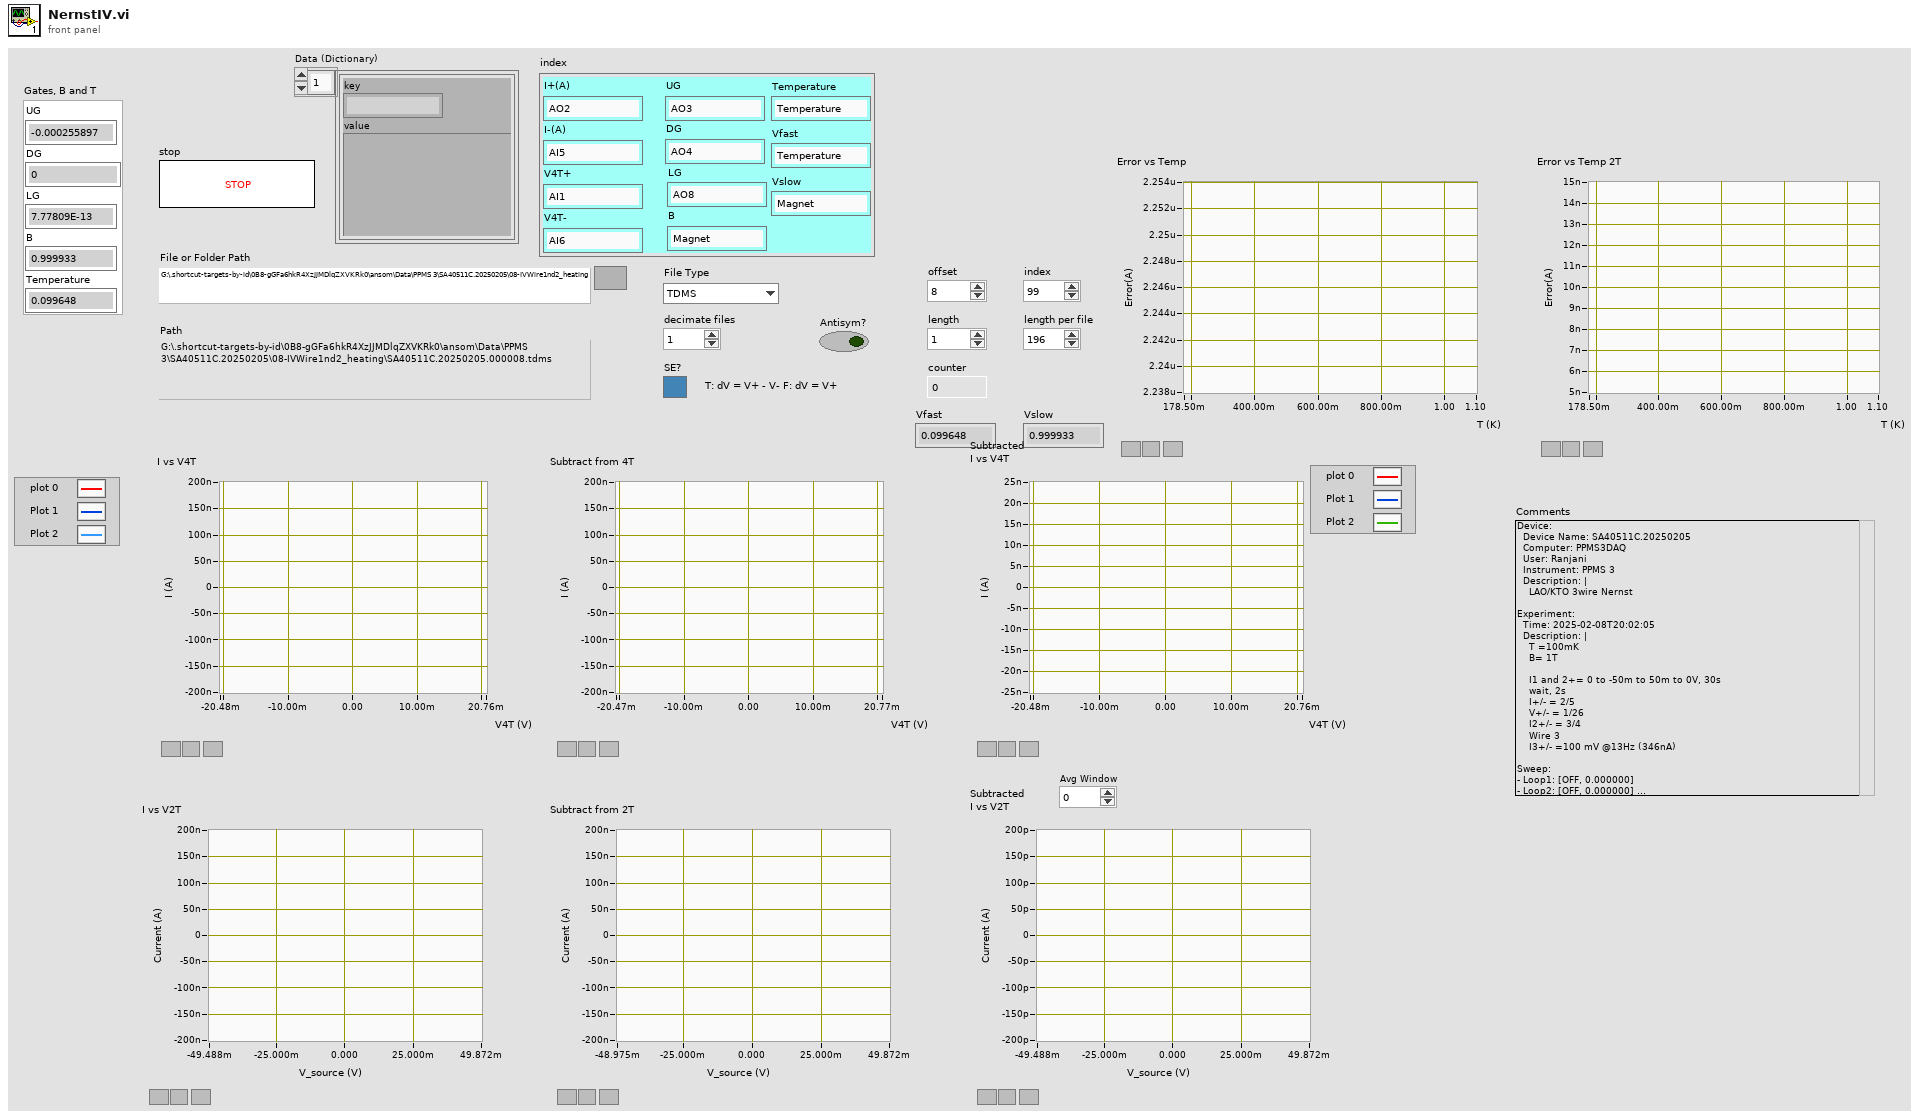
[diagram p1: front panel]
types:
  T1 = typedef "LV-Data.lvclass/File Type--enum.ctl" = enum16{"DAT", "ITX", "TDMS", "VI"}
  T2 = cluster{"I+(A)":string, "I-(A)":string, "V4T+":string, "V4T-":string, "UG":string, "DG":string, "LG":string, "B":string, "Temperature":string, "Vfast":string, "Vslow":string}
  T3 = typedef "LV-Data.lvclass/Dictionary--cluster.ctl" = cluster{"key":string, "value":variant}
  T4 = cluster{"UG":dbl, "DG":dbl, "LG":dbl, "B":dbl, "Temperature":dbl}
  T5 = typedef "Dictionary Object RefNum__ogtk.ctl" = refnum<k1>
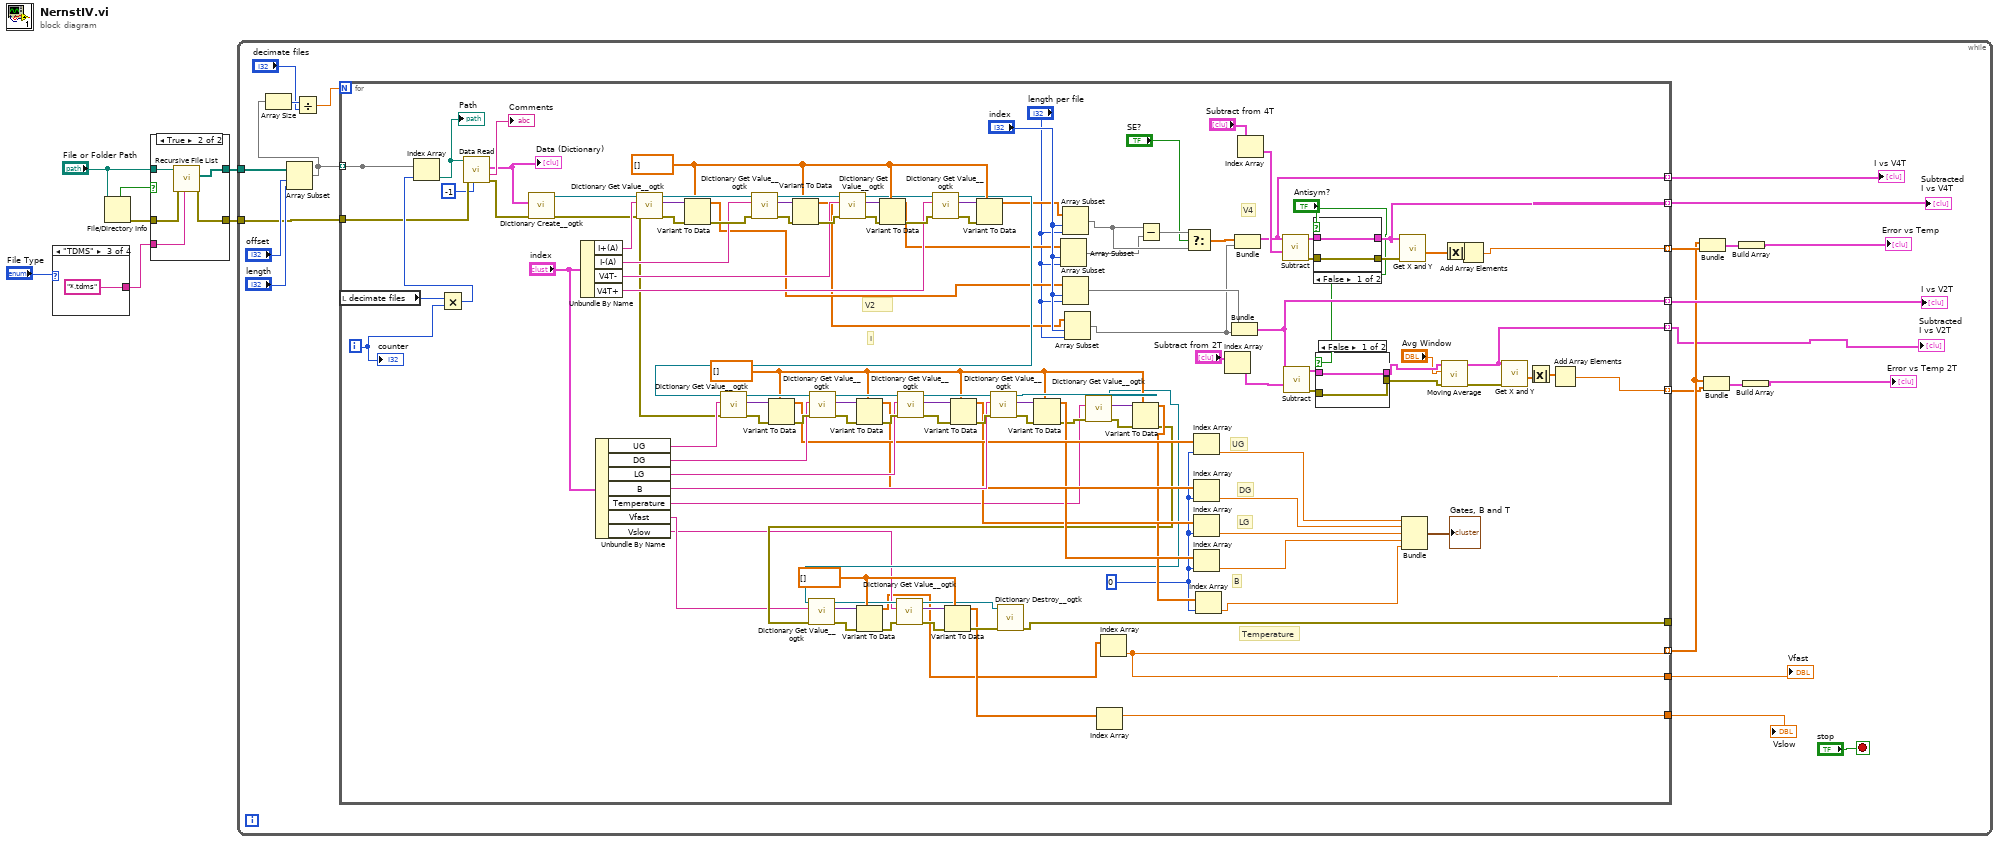
[diagram p0: block diagram]
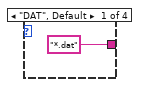
[diagram p2: hidden frame]
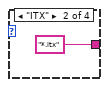
[diagram p3: hidden frame]
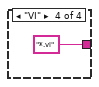
[diagram p4: hidden frame]
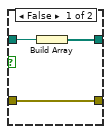
[diagram p5: hidden frame]
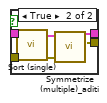
[diagram p6: hidden frame]
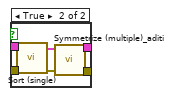
[diagram p7: hidden frame]
diagram:
  n1 = case shown="\"TDMS\"" "File Type" {
    tunnel: ["*.dat" ("pattern") "*.itx" ("pattern") "*.tdms" ("pattern") "*.vi" ("pattern")] -> w1
    frame "DAT", Default {
    }
    frame "ITX" {
    }
    frame "TDMS" {
    }
    frame "VI" {
    }
  }
  n2 = File/Directory Info(path="File or Folder Path") -> (directory=w5:bool, error out=w3:errorcluster)  [unwired: 1 in, 5 out]
  n3 = case shown="True" w5 {
    tunnel: [w14 w15] -> w6
    tunnel: "File or Folder Path" -> [w13 w19]
    tunnel: [w12 w18] -> w4
    tunnel: w3 -> [w12 w17]
    tunnel: w1 -> [_ w16]
    frame False {
      n4 = Build Array(w13) -> (w14:path[])
    }
    frame True {
      n5 = call <vilib>:"Recursive File List.vi"("pattern"=w16, "error in (no error)"=w17, "Folder Path"=w19) -> ("error out"=w18:errorcluster, "All Files in Dir"=w15:path[])  [unwired: 4 in, 3 out]
    }
  }
  n6 = while {
    tunnel: w6 -> [w39]
    tunnel: w4 -> [w34]
    stop <- "stop" stop-if-true
    n7 = Array Subset(array=w39, index="offset", length="length") -> (w35:path[])
    n8 = Array Size(array=w35) -> (size(s)=w38:i32)
    n9 = Divide(x=w38, y="decimate files") -> (x/y=w36:dbl)
    n10 = for {
      N: w36 -> [_]
      tunnel: w35 -> [w165]
      tunnel: [w165] -> _ mode=indexing
      tunnel: w34 -> [w160]
      tunnel: [w72] -> w30 mode=indexing
      tunnel: [w56] -> w31 mode=indexing
      tunnel: [w48] -> w25
      tunnel: [w79] -> w32
      tunnel: [w77] -> _
      tunnel: [w75] -> w29 mode=indexing
      tunnel: [w45] -> w20 mode=indexing
      tunnel: [w49] -> w26 mode=indexing
      tunnel: [w48] -> w23 mode=indexing
      tunnel: [w47] -> w22 mode=indexing
      i -> [w162]
      w94 = dbl[] []
      w95 = 0 ("index")
      w102 = dbl[] []
      w141 = dbl[] []
      # "Temperature"
      # "V4"
      # "I"
      # "V2"
      # "B"
      # "LG"
      # "DG"
      # "UG"
      n11 = local read "decimate files"() -> (w163:i32)
      n12 = Multiply(x=w163, y=w162) -> (x*y=w164:i32)
      n13 = Index Array(array=w165, index=w164) -> (element=w158:path)
      "Path" <- w158
      n14 = call <userlib>:"Data Read.vi"("Append Index"=-1, "error in (no error)"=w160, "path"=w158) -> ("error out"=w146:errorcluster, "Notes"=→"Comments":string, "Data (Dictionary)"=w157:T3[])  [unwired: 5 in, 1 out]
      "Data (Dictionary)" <- w157
      n15 = call <userlib>:"Dictionary Create__ogtk.vi"("error in (no error)"=w146, "initial dictionary (empty)"=w157) -> ("error out"=w105:errorcluster, "dictionary out"=w108:T5)  [unwired: 8 in]
      n16 = Unbundle By Name("index") -> ("I+(A)"=w156:string, "I-(A)"=w140:string, "V4T-"=w139:string, "V4T+"=w138:string)
      n17 = Unbundle By Name("index") -> ("UG"=w121:string, "DG"=w120:string, "LG"=w119:string, "B"=w118:string, "Temperature"=w99:string, "Vfast"=w83:string, "Vslow"=w82:string)
      n18 = call <userlib>:"Dictionary Get Value__ogtk.vi"("error in"=w105, "key"=w156, "dictionary"=w108) -> ("error out"=w145:errorcluster, "value"=w155:variant, "dictionary out"=w148:T5)  [unwired: 5 in, 1 out]
      n19 = Variant To Data(error in=w145, type=w141, Variant=w155) -> (data=w67:dbl[], error out=w144:errorcluster)
      n20 = call <userlib>:"Dictionary Get Value__ogtk.vi"("error in"=w144, "key"=w140, "dictionary"=w148) -> ("error out"=w150:errorcluster, "value"=w149:variant, "dictionary out"=w147:T5)  [unwired: 5 in, 1 out]
      n21 = Variant To Data(error in=w150, type=w141, Variant=w149) -> (data=w65:dbl[], error out=w143:errorcluster)
      n22 = call <userlib>:"Dictionary Get Value__ogtk.vi"("error in"=w143, "key"=w139, "dictionary"=w147) -> ("error out"=w154:errorcluster, "value"=w153:variant, "dictionary out"=w113:T5)  [unwired: 5 in, 1 out]
      n23 = Variant To Data(error in=w154, type=w141, Variant=w153) -> (data=w62:dbl[], error out=w142:errorcluster)
      n24 = call <userlib>:"Dictionary Get Value__ogtk.vi"("error in"=w142, "key"=w138, "dictionary"=w113) -> ("error out"=w152:errorcluster, "value"=w151:variant, "dictionary out"=w106:T5)  [unwired: 5 in, 1 out]
      n25 = call <userlib>:"Dictionary Get Value__ogtk.vi"("error in"=w105, "key"=w121, "dictionary"=w106) -> ("error out"=w125:errorcluster, "value"=w135:variant, "dictionary out"=w128:T5)  [unwired: 5 in, 1 out]
      n26 = Variant To Data(error in=w125, type=w102, Variant=w135) -> (data=w116:dbl[], error out=w124:errorcluster)
      n27 = call <userlib>:"Dictionary Get Value__ogtk.vi"("error in"=w124, "key"=w120, "dictionary"=w128) -> ("error out"=w130:errorcluster, "value"=w129:variant, "dictionary out"=w127:T5)  [unwired: 5 in, 1 out]
      n28 = Variant To Data(error in=w130, type=w102, Variant=w129) -> (data=w115:dbl[], error out=w123:errorcluster)
      n29 = call <userlib>:"Dictionary Get Value__ogtk.vi"("error in"=w123, "key"=w119, "dictionary"=w127) -> ("error out"=w134:errorcluster, "value"=w133:variant, "dictionary out"=w126:T5)  [unwired: 5 in, 1 out]
      n30 = Variant To Data(error in=w134, type=w102, Variant=w133) -> (data=w107:dbl[], error out=w122:errorcluster)
      n31 = Variant To Data(error in=w152, type=w141, Variant=w151) -> (data=w64:dbl[])  [unwired: 1 out]
      n32 = call <userlib>:"Dictionary Get Value__ogtk.vi"("error in"=w122, "key"=w118, "dictionary"=w126) -> ("error out"=w132:errorcluster, "value"=w131:variant, "dictionary out"=w117:T5)  [unwired: 5 in, 1 out]
      n33 = Variant To Data(error in=w132, type=w102, Variant=w131) -> (data=w114:dbl[], error out=w100:errorcluster)
      n34 = Array Subset(array=w62, index="index", length="length per file") -> (w61:dbl[])
      n35 = Array Subset(array=w64, index="index", length="length per file") -> (w63:dbl[])
      n36 = Array Subset(array=w67, index="index", length="length per file") -> (w66:dbl[])
      n37 = Array Subset(array=w65, index="index", length="length per file") -> (w59:dbl[])
      n38 = call <userlib>:"Dictionary Get Value__ogtk.vi"("error in"=w100, "key"=w99, "dictionary"=w117) -> ("error out"=w101:errorcluster, "value"=w103:variant, "dictionary out"=w85:T5)  [unwired: 5 in, 1 out]
      n39 = Variant To Data(error in=w101, type=w102, Variant=w103) -> (data=w98:dbl[], error out=w84:errorcluster)
      n40 = call <userlib>:"Dictionary Get Value__ogtk.vi"("error in"=w84, "key"=w83, "dictionary"=w85) -> ("error out"=w92:errorcluster, "value"=w88:variant, "dictionary out"=w91:T5)  [unwired: 5 in, 1 out]
      n41 = Variant To Data(error in=w92, type=w94, Variant=w88) -> (data=w80:dbl[], error out=w93:errorcluster)
      n42 = call <userlib>:"Dictionary Get Value__ogtk.vi"("error in"=w93, "key"=w82, "dictionary"=w91) -> ("error out"=w89:errorcluster, "value"=w90:variant, "dictionary out"=w86:T5)  [unwired: 5 in, 1 out]
      n43 = Variant To Data(error in=w89, type=w94, Variant=w90) -> (data=w81:dbl[], error out=w87:errorcluster)
      n44 = call <userlib>:"Dictionary Destroy__ogtk.vi"("error in (no error)"=w87, "dictionary"=w86) -> ("error out"=w77:errorcluster)  [unwired: 9 in]
      n45 = Index Array(array=w81) -> (element=w79:dbl)  [unwired: 1 in]
      n46 = Index Array(array=w80) -> (element=w48:dbl)  [unwired: 1 in]
      n47 = Subtract(x=w63, y=w61) -> (x-y=w137:dbl[])
      n48 = Select(t=w137, s="SE?", f=w63) -> (s? t:f=w78:dbl[])
      n49 = Index Array(array=w116, index=w95) -> (element=w112:dbl)
      n50 = Index Array(array=w115, index=w95) -> (element=w110:dbl)
      n51 = Index Array(array=w107, index=w95) -> (element=w111:dbl)
      n52 = Index Array(array=w114, index=w95) -> (element=w109:dbl)
      n53 = Index Array(array=w98, index=w95) -> (element=w97:dbl)
      n54 = Index Array(array="Subtract from 2T") -> (element=w73:cluster{dbl[], dbl[]})  [unwired: 1 in]
      n55 = Bundle(w66, w59) -> (w72:cluster{dbl[], dbl[]})  [unwired: 1 in]
      n56 = Bundle(w78, w59) -> (w75:cluster{dbl[], dbl[]})  [unwired: 1 in]
      n57 = Index Array(array="Subtract from 4T") -> (element=w76:cluster{dbl[], dbl[]})  [unwired: 1 in]
      n58 = call-poly <userlib>:"Subtract.vi"("y"=w76, "XY-data"=w75) -> ("error out"=w57:errorcluster, "XY-data out"=w58:cluster{"X-array":dbl[], "Y-array":dbl[]})  [unwired: 8 in]
      n59 = call-poly <userlib>:"Subtract.vi"("y"=w73, "XY-data"=w72) -> ("error out"=w52:errorcluster, "XY-data out"=w53:cluster{"X-array":dbl[], "Y-array":dbl[]})  [unwired: 8 in]
      n60 = case shown="False" "Antisym?" {
        tunnel: w58 -> [w174 w181]
        tunnel: w57 -> [w175 w180]
        tunnel: [w174 w177] -> w56
        tunnel: [w175 w176] -> w55
        frame False {
        }
        frame True {
          n61 = call <userlib>:"Sort (single).vi"("error in (no error)"=w180, "XY-data"=w181) -> ("error out"=w178:errorcluster, "Sorted XY-data out"=w179:cluster{"X-array":dbl[], "Y-array":dbl[]})  [unwired: 7 in, 1 out]
          n62 = call "Symmetrize (multiple)_aditi.vi"("error in (no error)"=w178, "XY-data"=w179) -> ("error out"=w176:errorcluster, "Antisymmetric"=w177:cluster{"X-array":dbl[], "Y-array":dbl[]})  [unwired: 6 in, 2 out]
        }
      }
      n63 = case shown="False" "Antisym?" {
        tunnel: w53 -> [w167 w173]
        tunnel: w52 -> [w166 w172]
        tunnel: [w167 w169] -> w46
        tunnel: [w166 w168] -> w43
        frame False {
        }
        frame True {
          n64 = call <userlib>:"Sort (single).vi"("error in (no error)"=w172, "XY-data"=w173) -> ("error out"=w170:errorcluster, "Sorted XY-data out"=w171:cluster{"X-array":dbl[], "Y-array":dbl[]})  [unwired: 7 in, 1 out]
          n65 = call "Symmetrize (multiple)_aditi.vi"("error in (no error)"=w170, "XY-data"=w171) -> ("error out"=w168:errorcluster, "Antisymmetric"=w169:cluster{"X-array":dbl[], "Y-array":dbl[]})  [unwired: 6 in, 2 out]
        }
      }
      n66 = call-poly <userlib>:"Get X and Y.vi"("error in (no error)"=w55, "XY-data"=w56) -> ("Y-array"=w69:dbl[])  [unwired: 6 in, 3 out]
      n67 = Bundle(w112, w110, w111, w109, w97) -> (→"Gates, B and T":cluster{dbl, dbl, dbl, dbl, dbl})  [unwired: 1 in]
      n68 = call-poly <userlib>:"Moving Average.vi"("error in (no error)"=w43, "Window"="Avg Window", "XY-data"=w46) -> ("error out"=w44:errorcluster, "XY-data out"=w45:cluster{"X-array":dbl[], "Y-array":dbl[]})  [unwired: 7 in]
      n69 = Absolute Value(x=w69) -> (abs(x)=w70:dbl[])
      n70 = Add Array Elements(numeric array=w70) -> (sum=w49:dbl)
      n71 = call-poly <userlib>:"Get X and Y.vi"("error in (no error)"=w44, "XY-data"=w45) -> ("Y-array"=w51:dbl[])  [unwired: 6 in, 3 out]
      n72 = Absolute Value(x=w51) -> (abs(x)=w50:dbl[])
      n73 = Add Array Elements(numeric array=w50) -> (sum=w47:dbl)
      "counter" <- w162
    }
    "I vs V2T" <- w30
    "Subtracted \nI vs V4T" <- w31
    "Vslow" <- w32
    "Vfast" <- w25
    "I vs V4T" <- w29
    "Subtracted\nI vs V2T" <- w20
    n74 = Bundle(w23, w26) -> (w28:cluster{dbl[], dbl[]})  [unwired: 1 in]
    n75 = Bundle(w23, w22) -> (w24:cluster{dbl[], dbl[]})  [unwired: 1 in]
    n76 = Build Array(w28) -> (→"Error vs Temp":cluster{dbl[], dbl[]}[])
    n77 = Build Array(w24) -> (→"Error vs Temp 2T":cluster{dbl[], dbl[]}[])
  }
